vi "Simon_Mouse.vi"() -> ()   [LabVIEW 2019]
uses:
  <vilib>/numeric/Random Number (Range) U64.vi
  <vilib>/numeric/sub_Random U32.vi
  <vilib>/Utility/file.llb/Write Delimited Spreadsheet (I64).vi
panel:
  in  "读档":bool
  in  "存档":bool
  in  "亮灯次数":i32=1
  out "难度：分数":string
  out "倒计时":i32(slide) scale=-1.0..3635.0
  in  "是否开始计时？":bool
  out "分数":i32
  out "难度":string="困难"
  out "闪烁间隔":i32=727
  out "超时时间":i32=500
  out "User name out":string
  in  "User name in":string
  in  "结束":bool
  out "时间到":bool
  out "上":bool
  out "左":bool
  out "右":bool
  out "下":bool
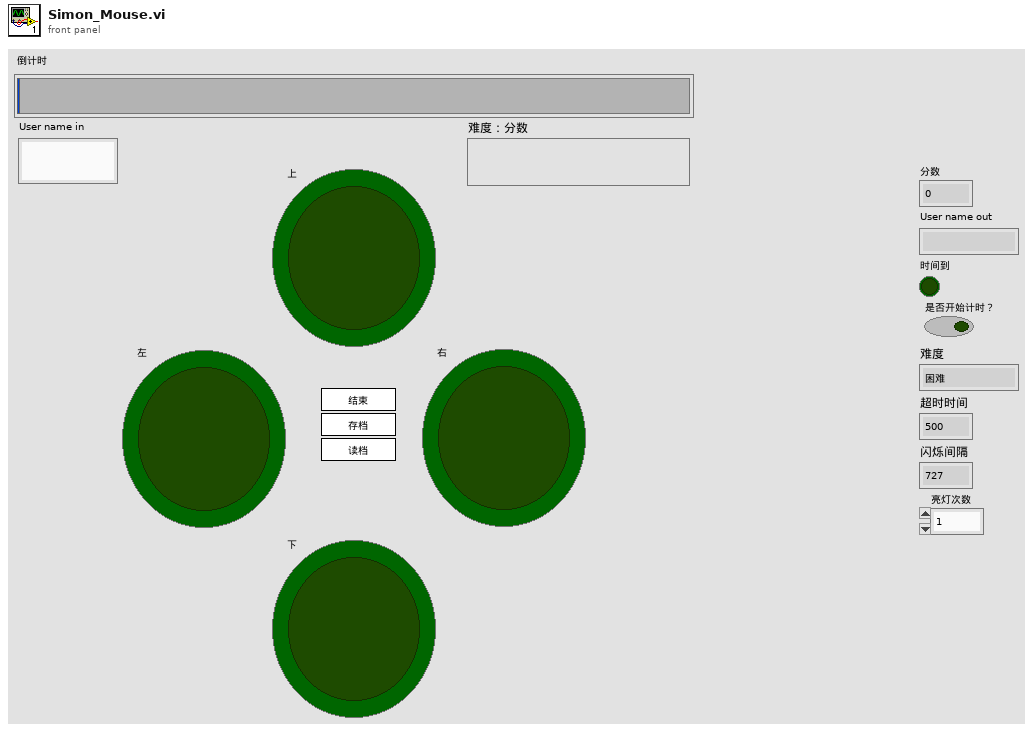
[diagram p1: front panel]
types:
  T1 = enum32{"Invalid", "Standard", "Closed", "Hidden", "Minimized", "Maximized"}
  T2 = enum32{"invalid app kind", "Development System", "Run Time System", "Student Edition", "Embedded LabVIEW", "Evaluation", "Custom"}
  T3 = typedef "按键枚举.ctl" = enum16{"读档", "存档", "按错", "退出", "黄", "红", "蓝", "绿"}
  T4 = cluster{"Core":cluster{"Current VI Reference":refnum<vi>, "Close Panel on Exit?":bool, "难度_保存":string, "亮灯次数_保存":i32, "超时时间_保存":i32, "闪烁间隔_保存":i32, "积分_保存":i32}}
  T5 = cluster{"Current VI Reference":refnum<vi>, "Close Panel on Exit?":bool, "难度_保存":string, "亮灯次数_保存":i32, "超时时间_保存":i32, "闪烁间隔_保存":i32, "积分_保存":i32}
  T6 = enum16{"Left Button", "Center Button", "Right Button", "Window Close"}
  T7 = typedef "eventvkey.ctl" = enum16{"ASCII", "Enter", "Return", "Shift", "Ctrl", "Alt", "Cmd", "Opt", "Caps", "NumLock", "Clear", "Break", "Up", "Down", "Left", "Right", "Insert", "Delete", "Home", "End", "PageUp", "PageDown", "Escape", "Help", "Pause", "ScrollLock", "F1", "F2", "F3", "F4", "F5", "F6", "F7", "F8", "F9", "F10", "F11", "F12", "F13", "F14", "F15", "F16", "F17", "F18", "F19", "F20", "F21", "F22", "F23", "F24", "Play", "VolumeUp", "VolumeDown", "Mute", "Two Byte Char"}
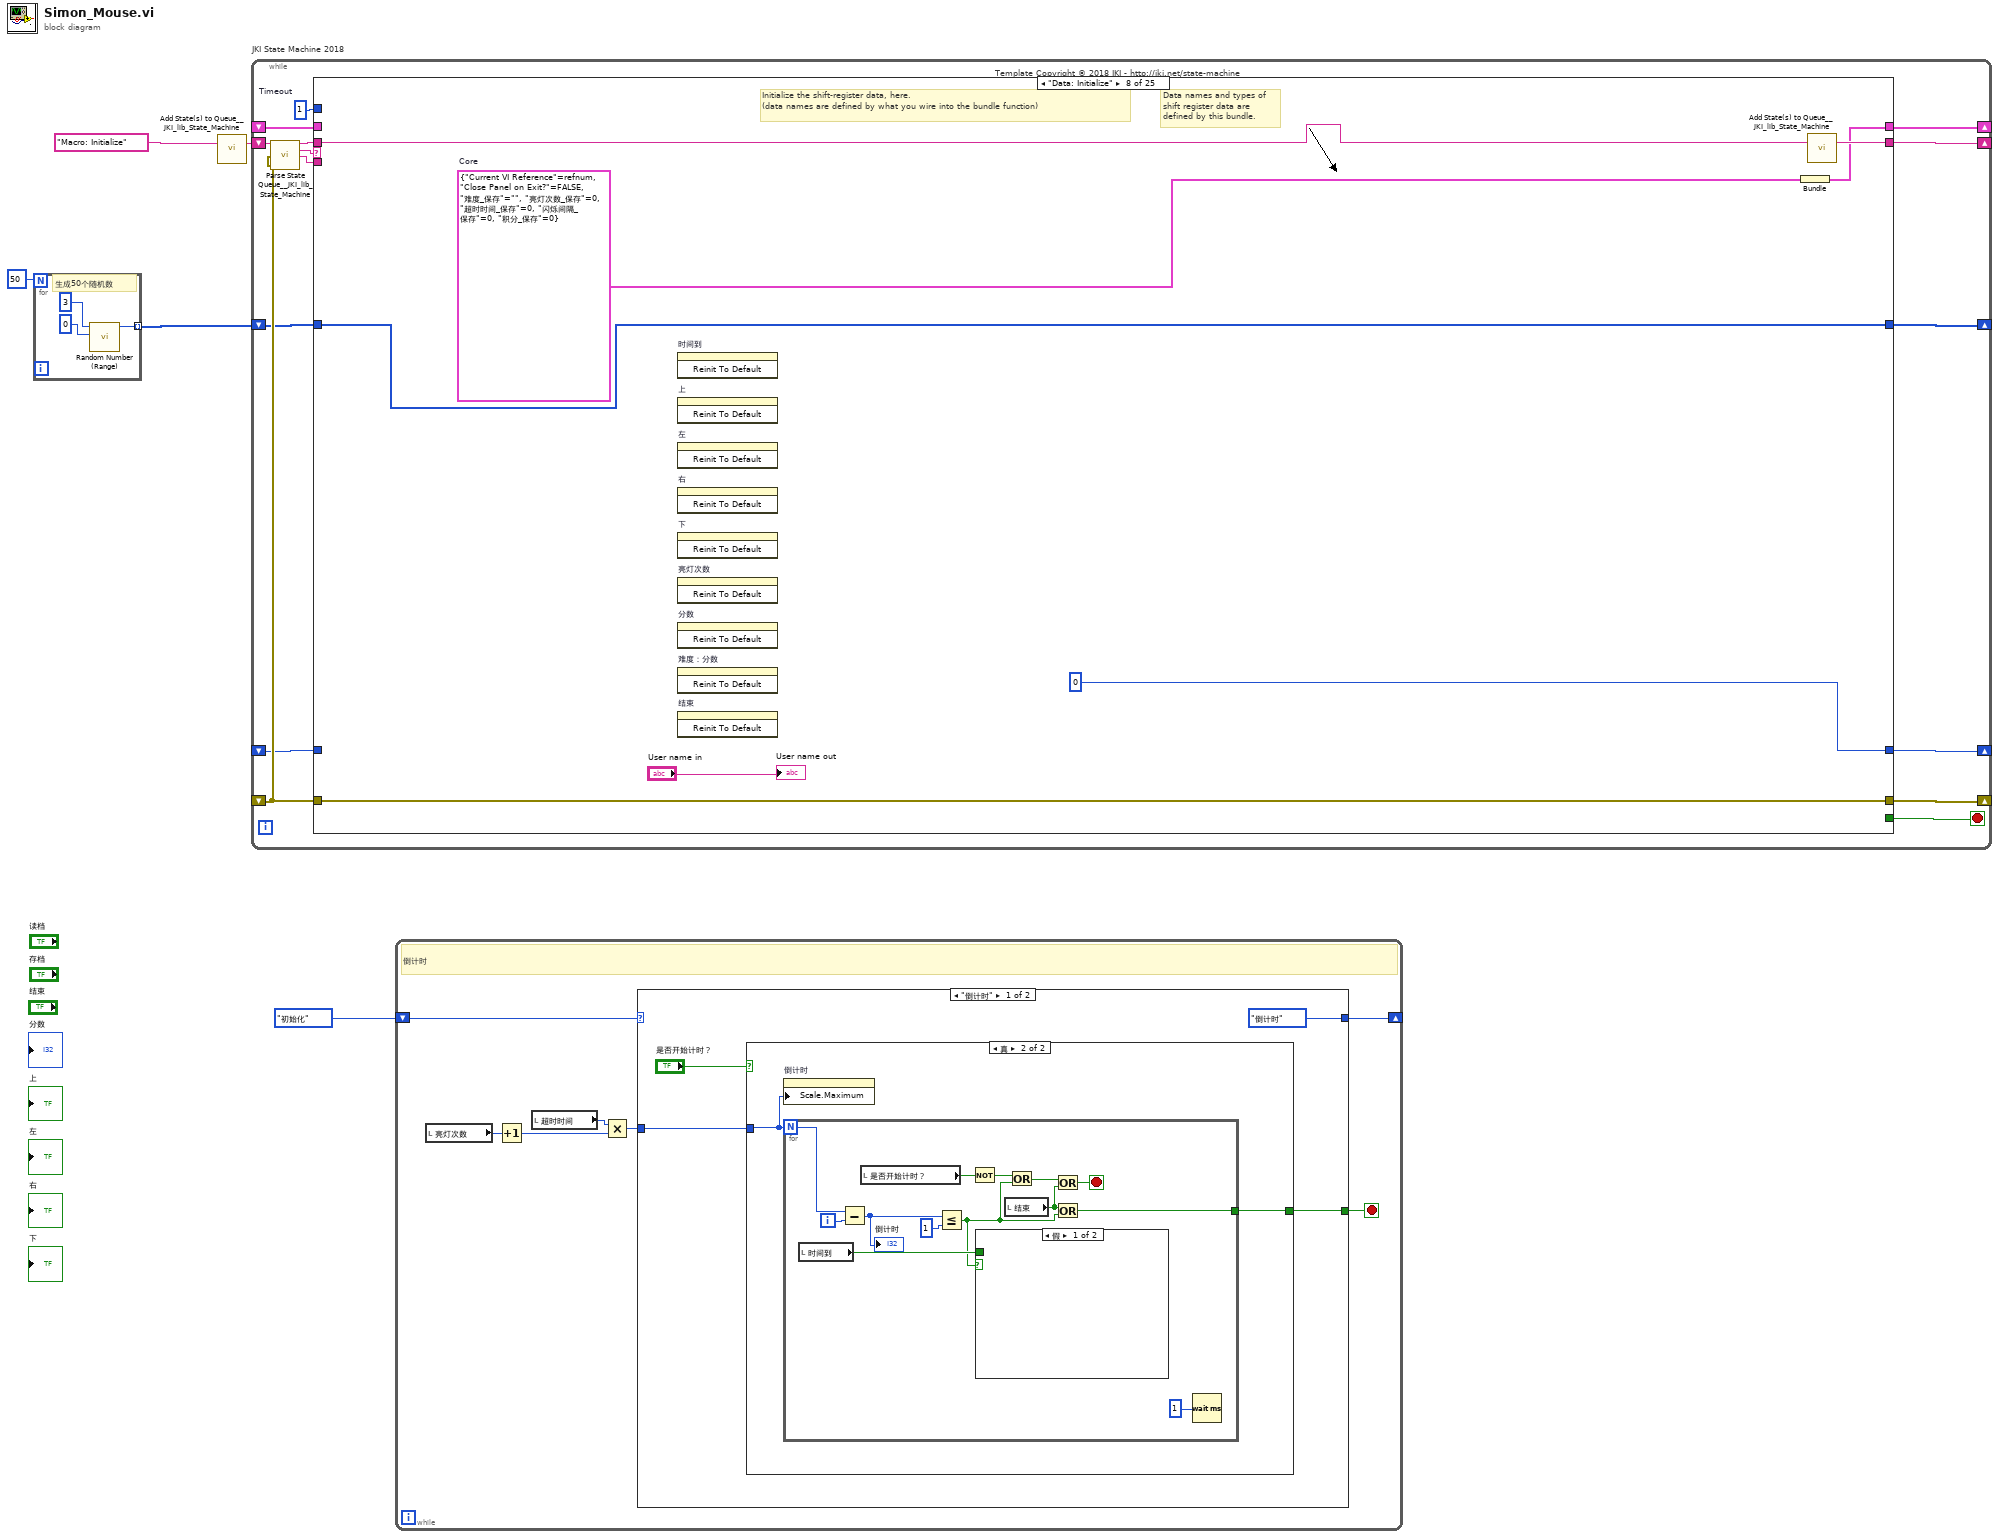
[diagram p0: block diagram]
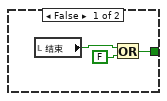
[diagram p2: hidden frame]
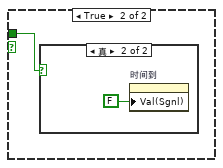
[diagram p3: hidden frame]
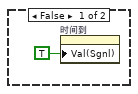
[diagram p4: hidden frame]
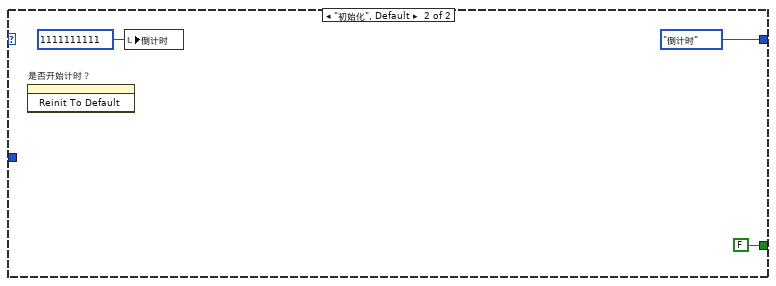
[diagram p5: hidden frame]
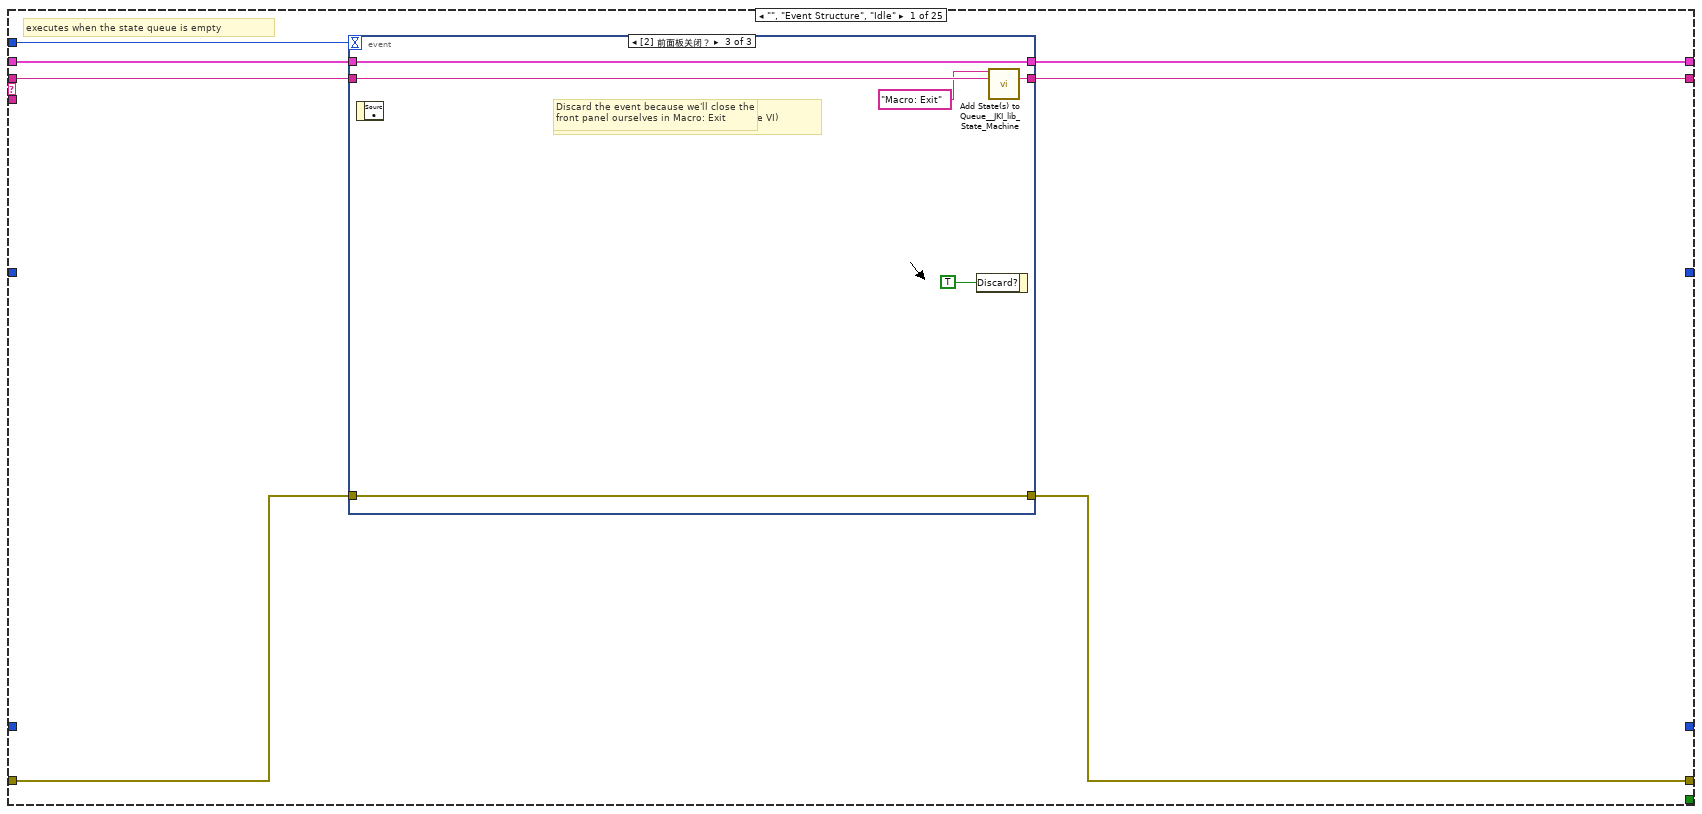
[diagram p6: hidden frame]
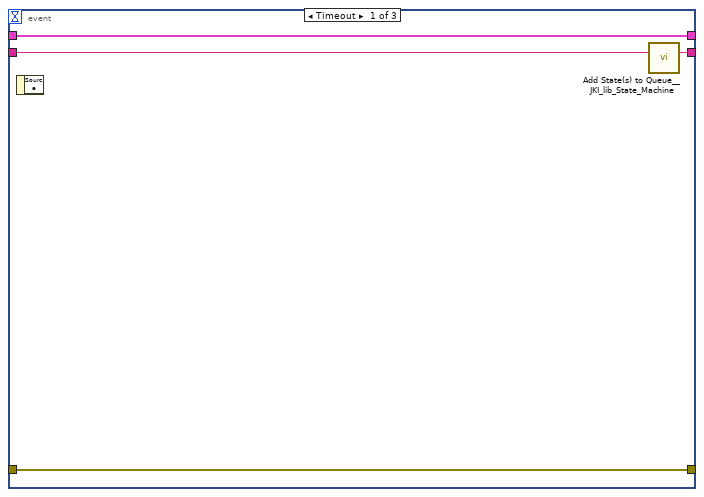
[diagram p7: hidden frame]
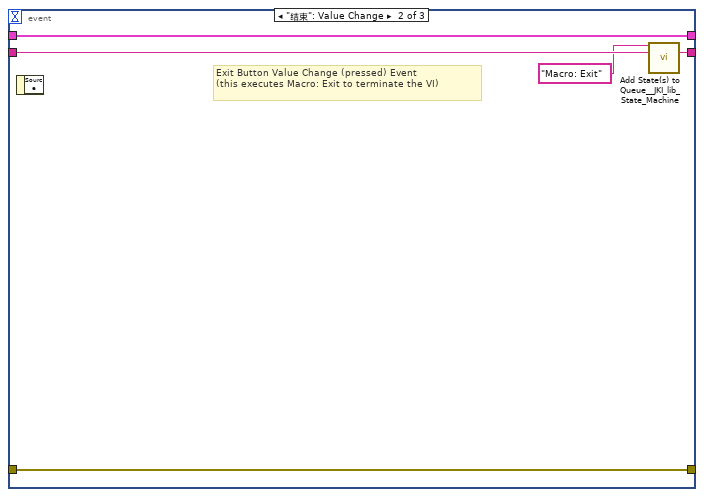
[diagram p8: hidden frame]
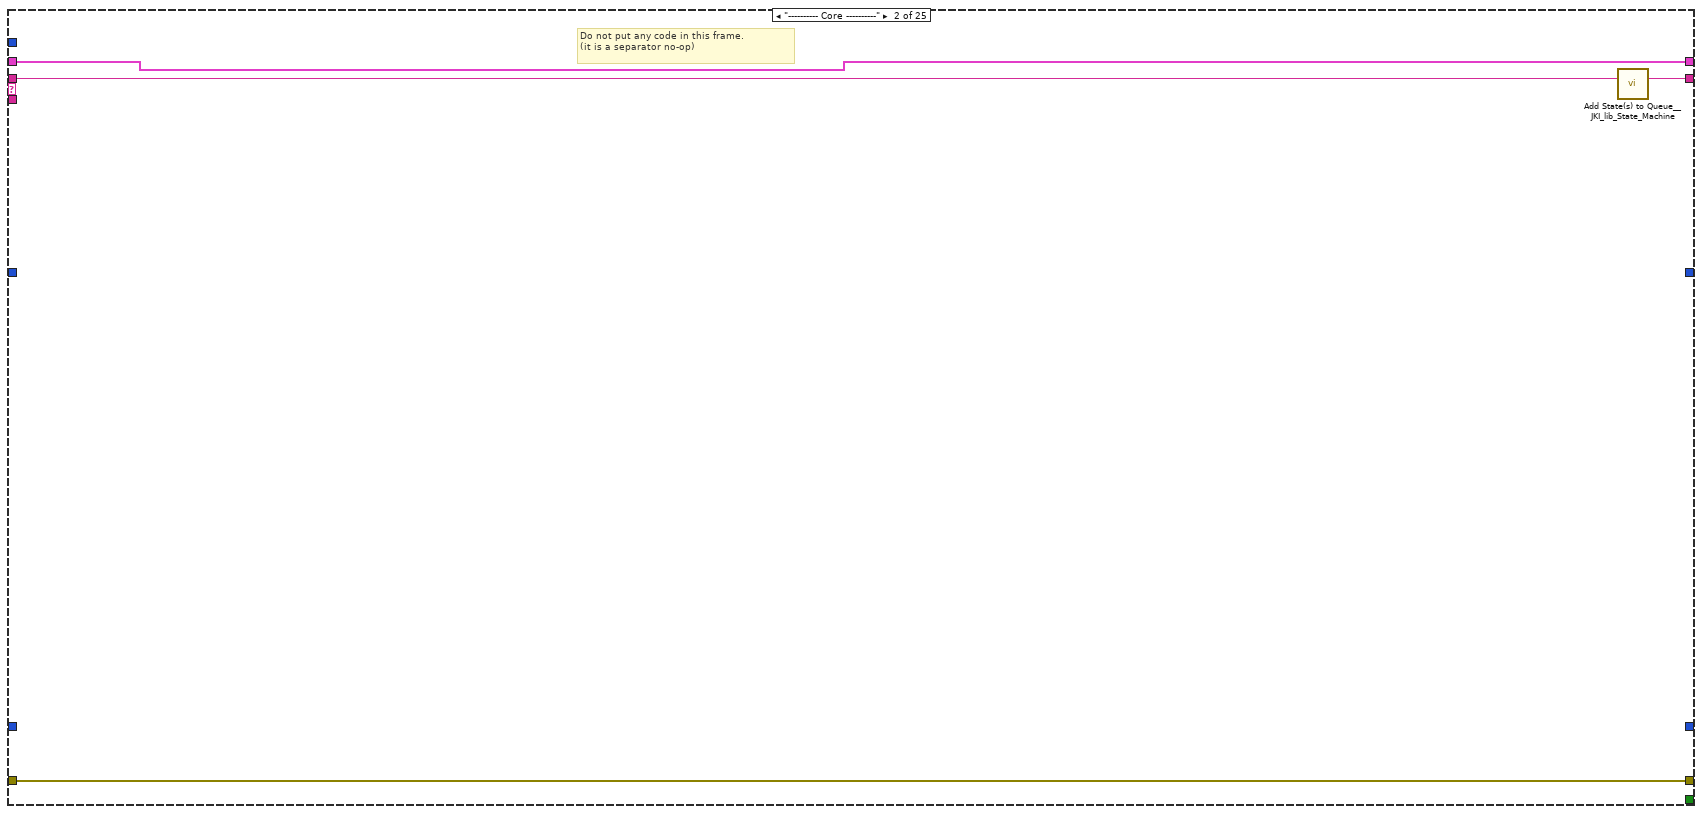
[diagram p9: hidden frame]
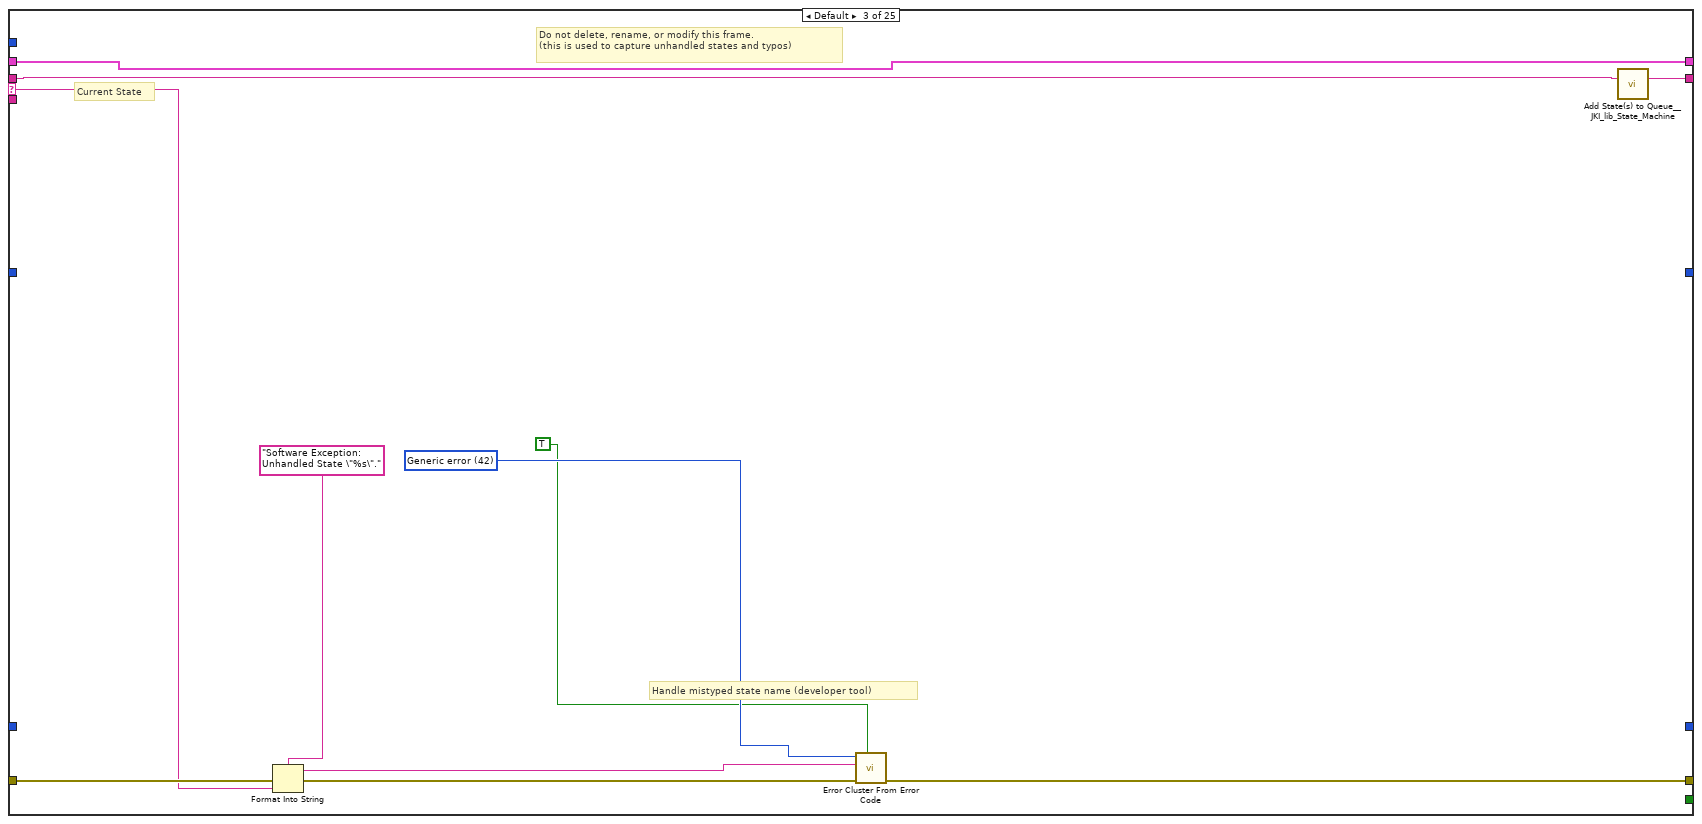
[diagram p10: hidden frame]
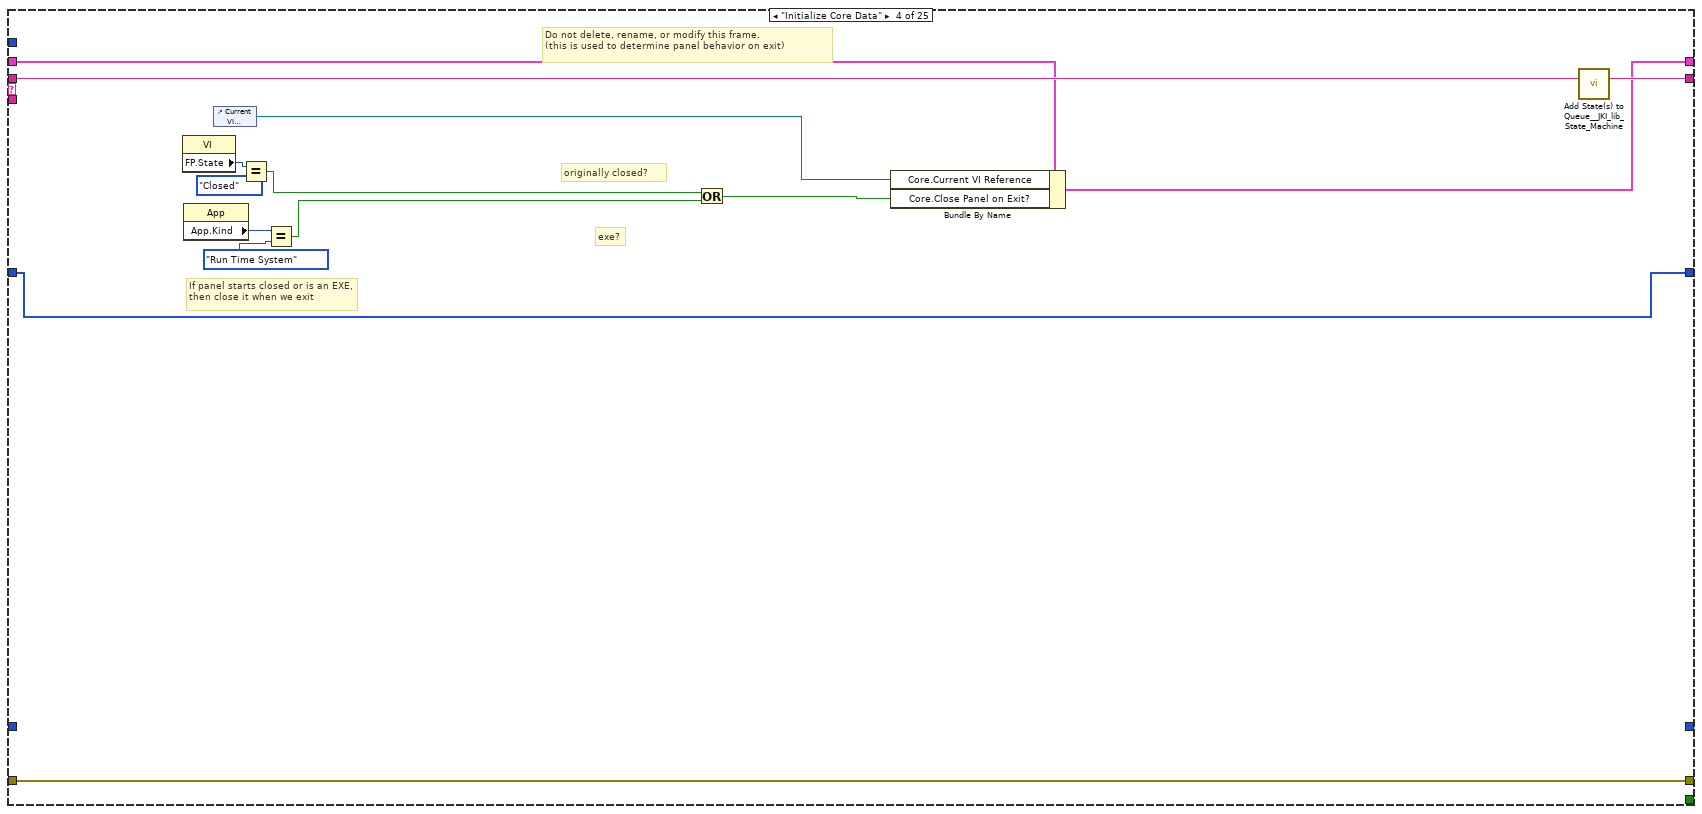
[diagram p11: hidden frame]
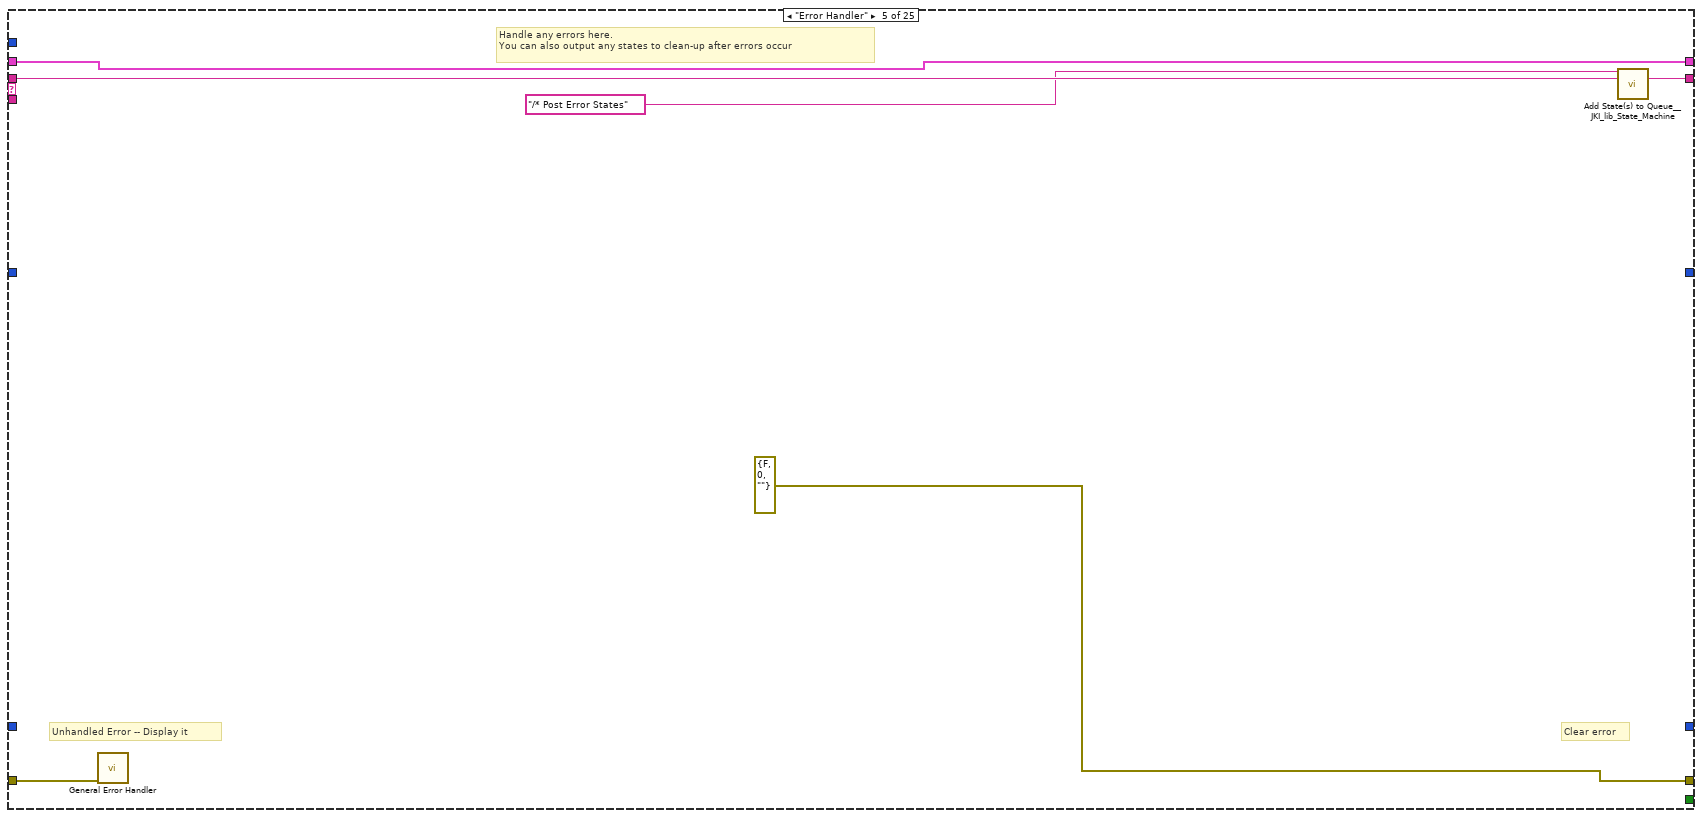
[diagram p12: hidden frame]
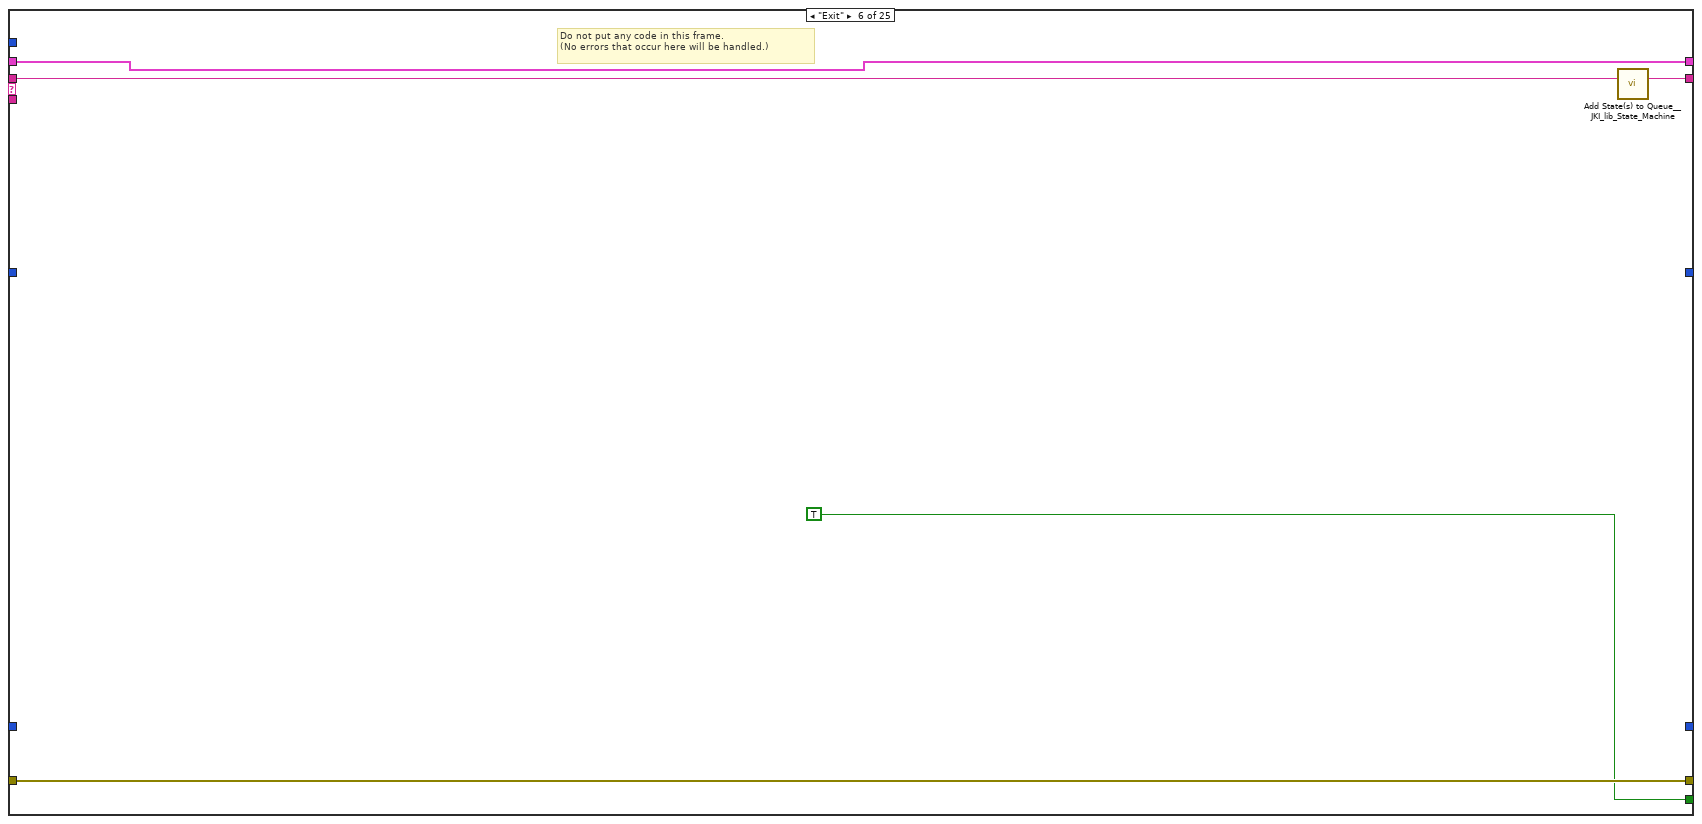
[diagram p13: hidden frame]
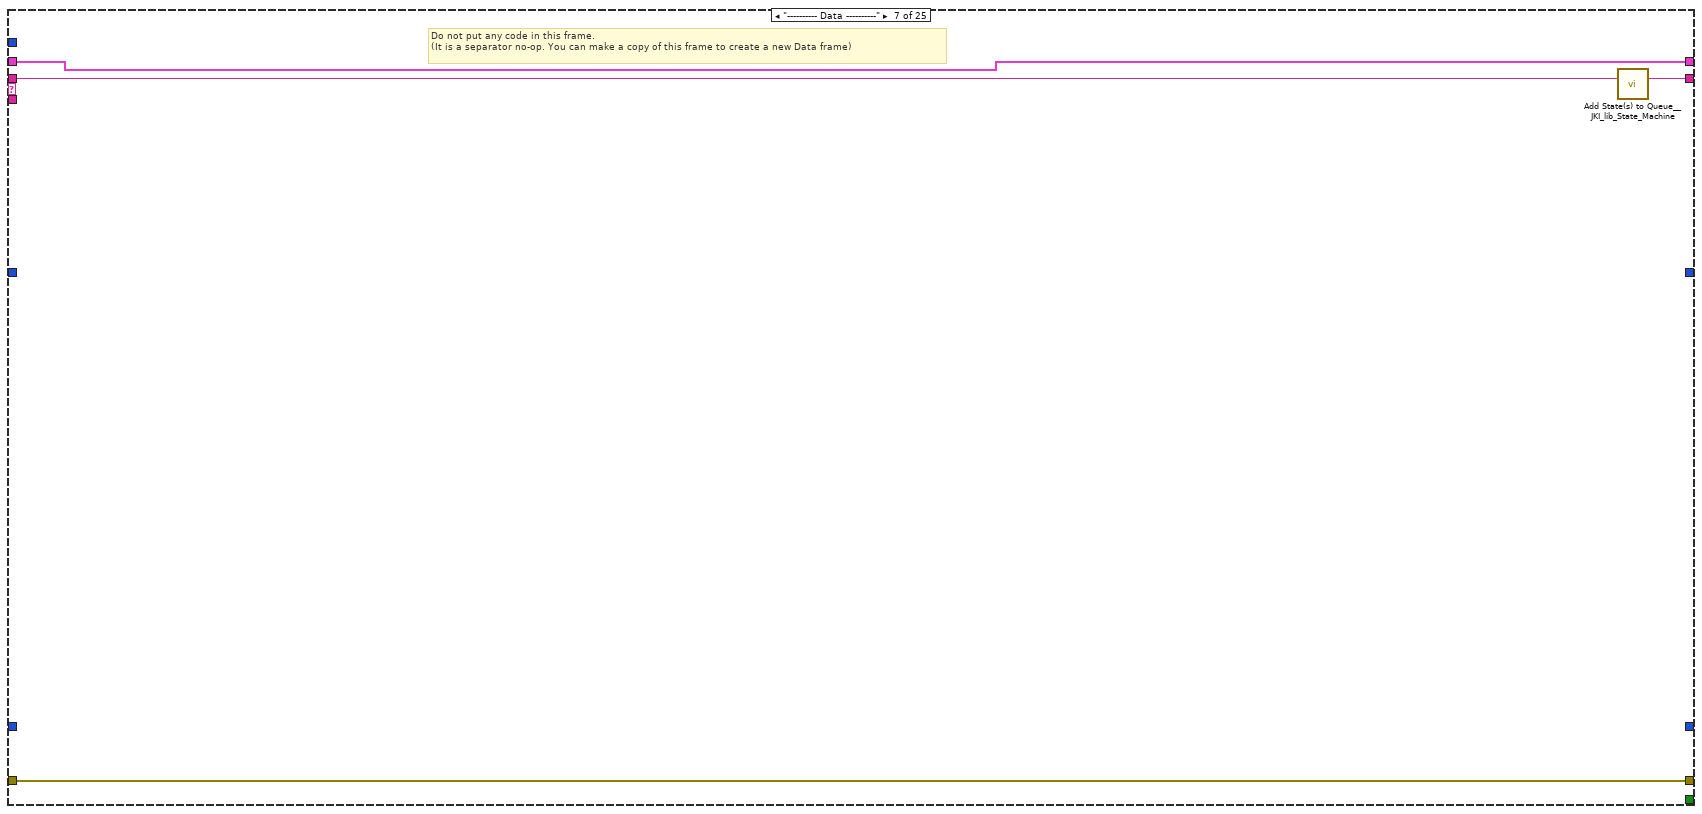
[diagram p14: hidden frame]
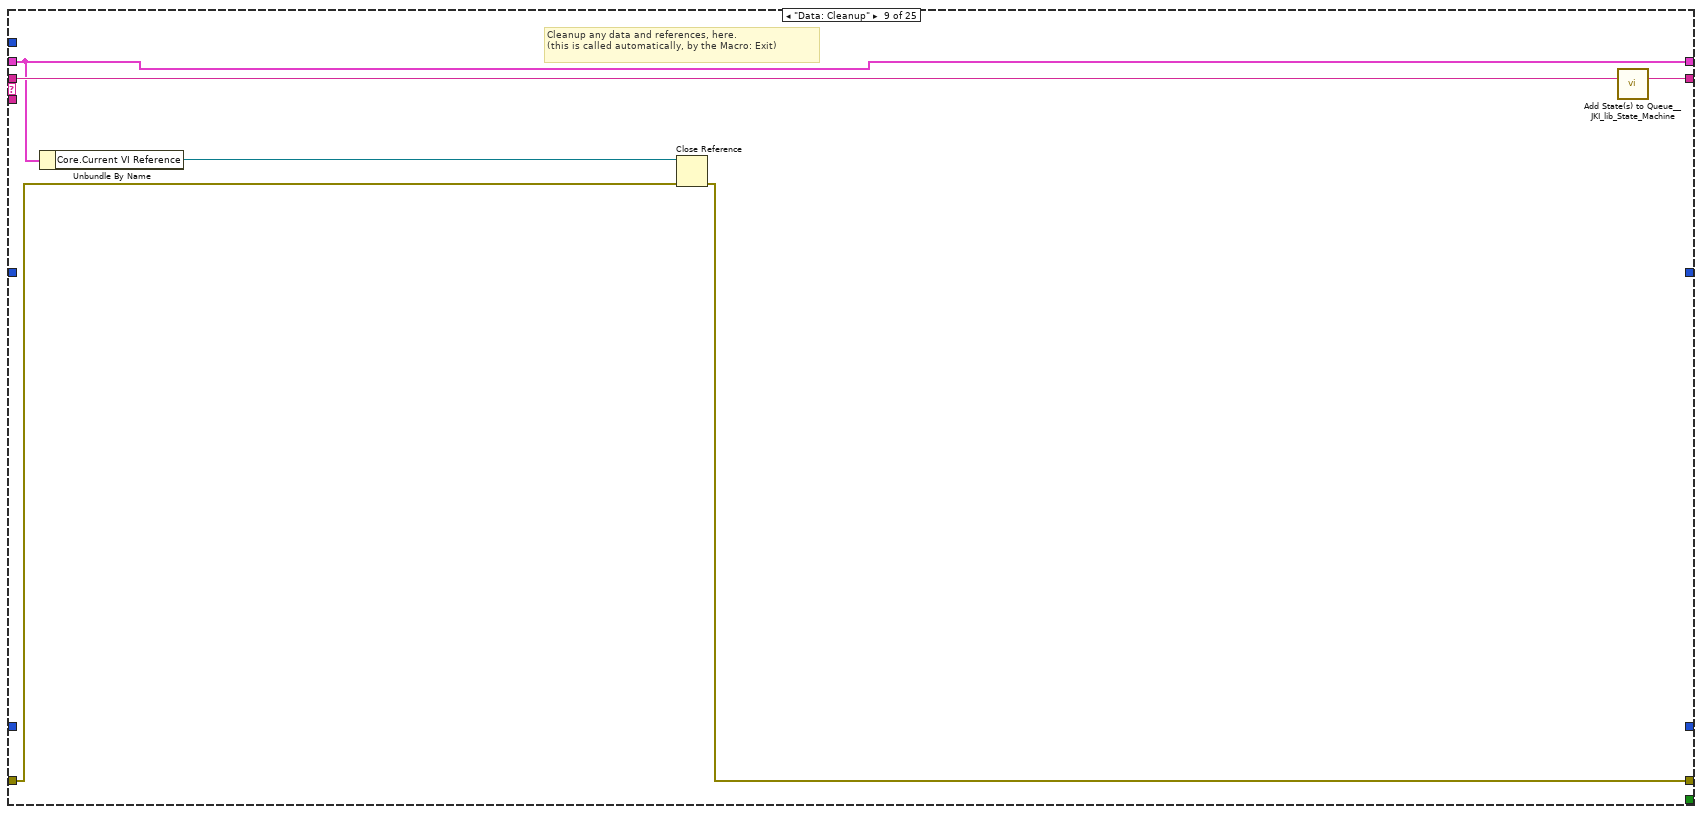
[diagram p15: hidden frame]
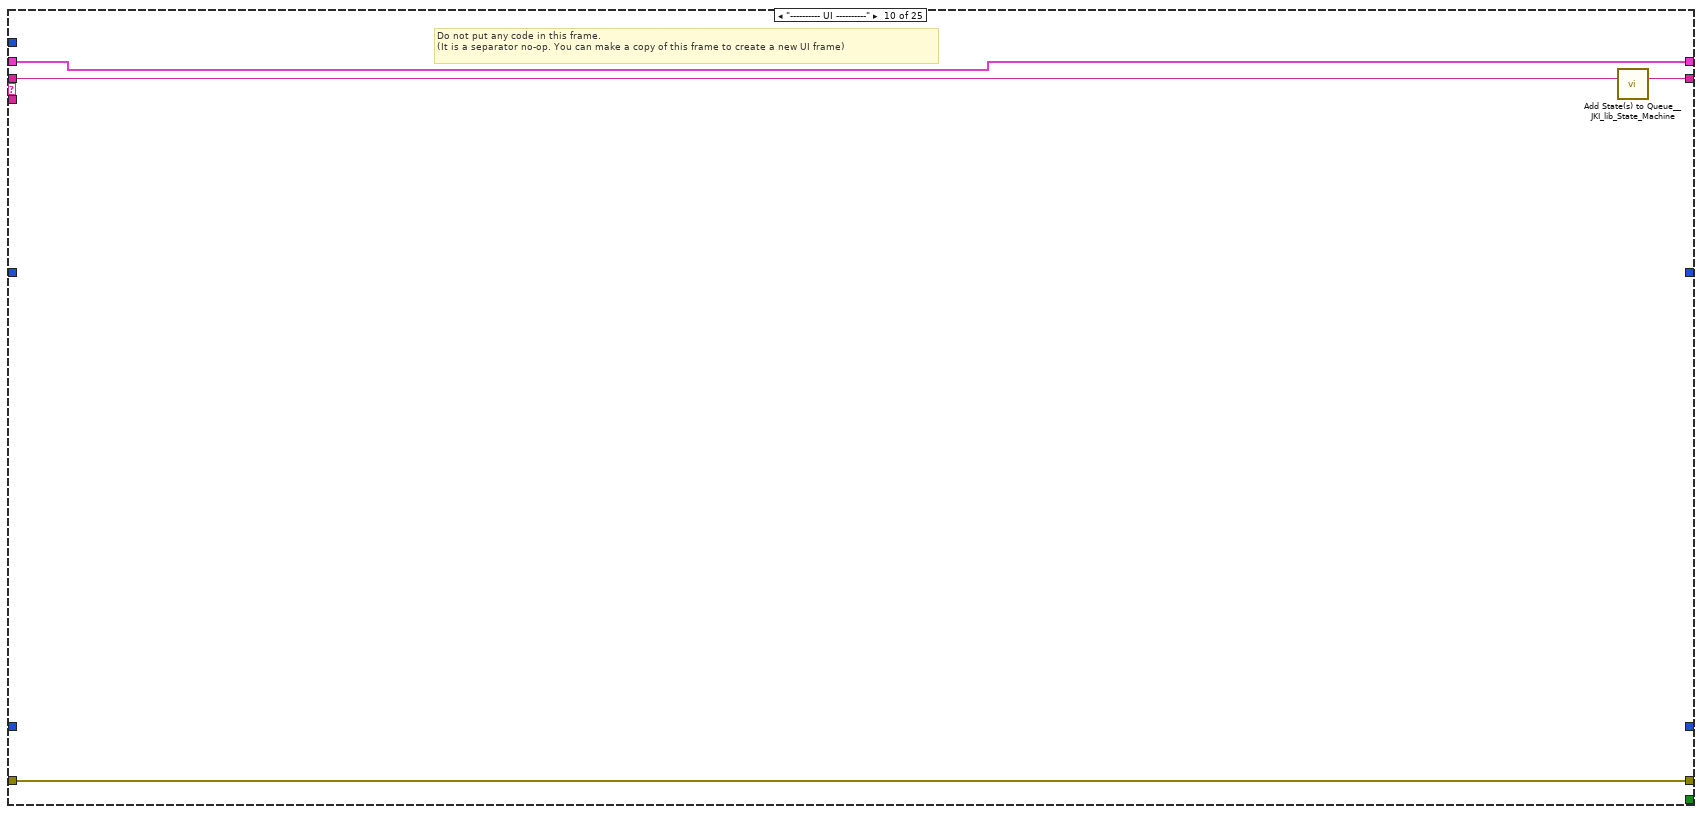
[diagram p16: hidden frame]
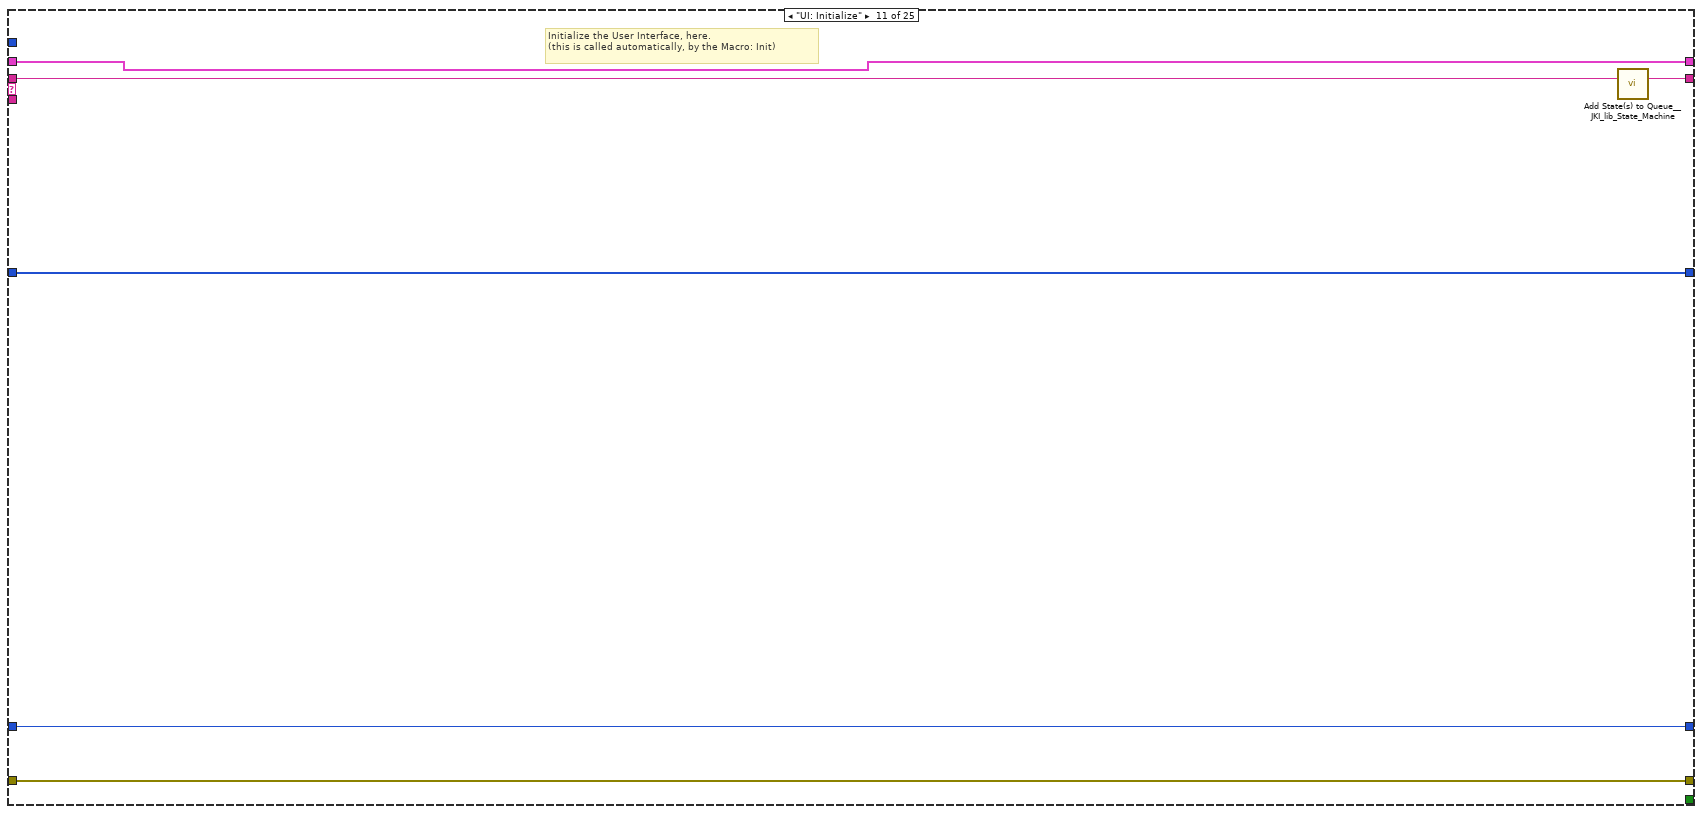
[diagram p17: hidden frame]
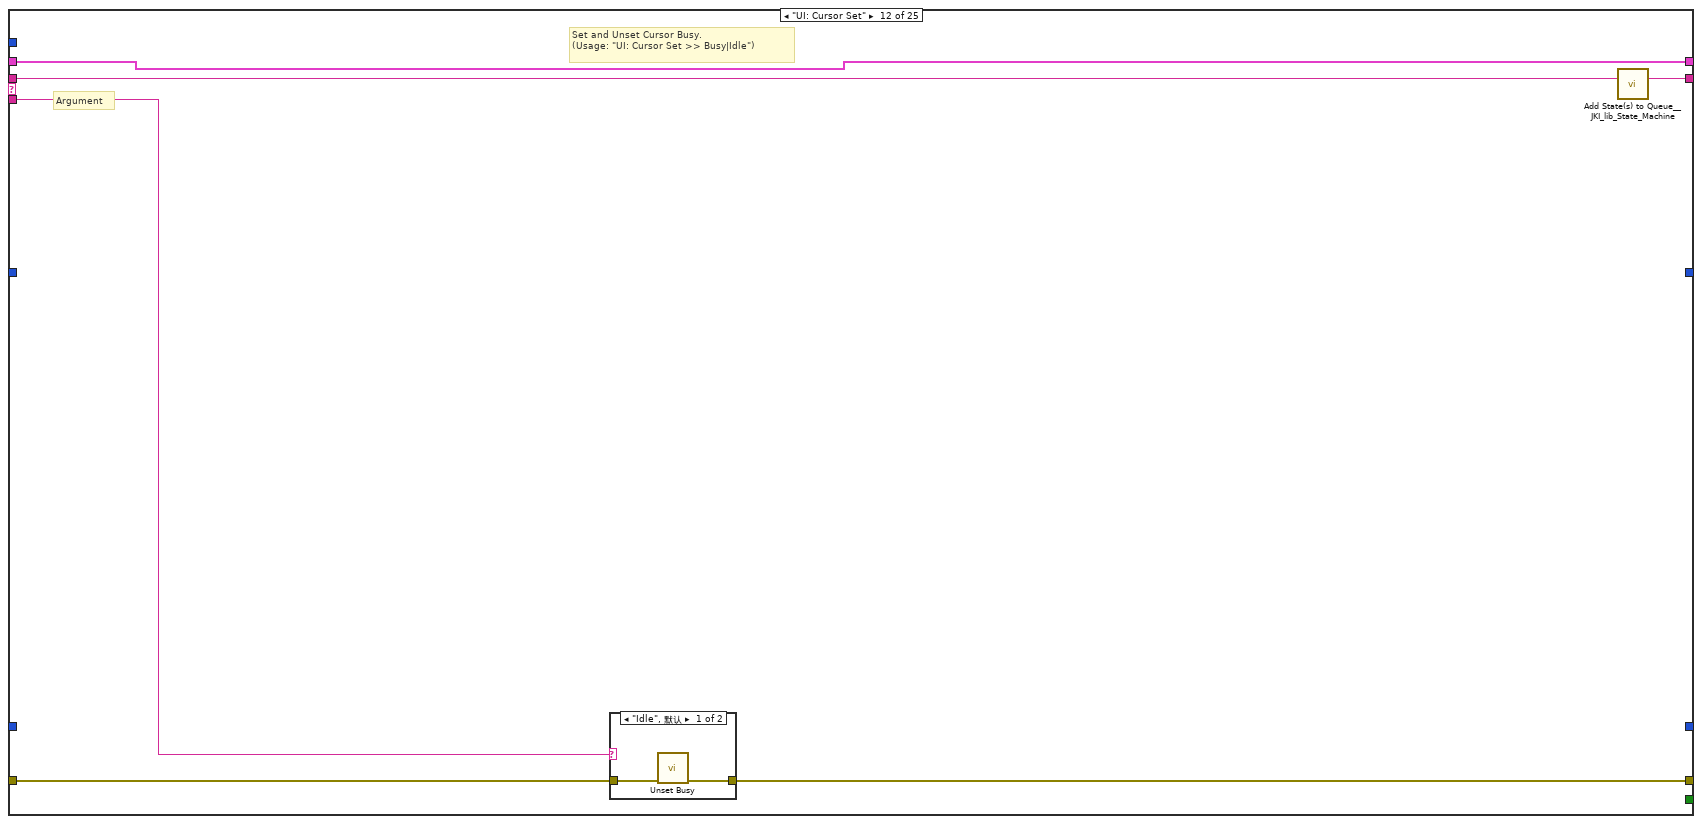
[diagram p18: hidden frame]
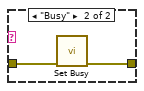
[diagram p19: hidden frame]
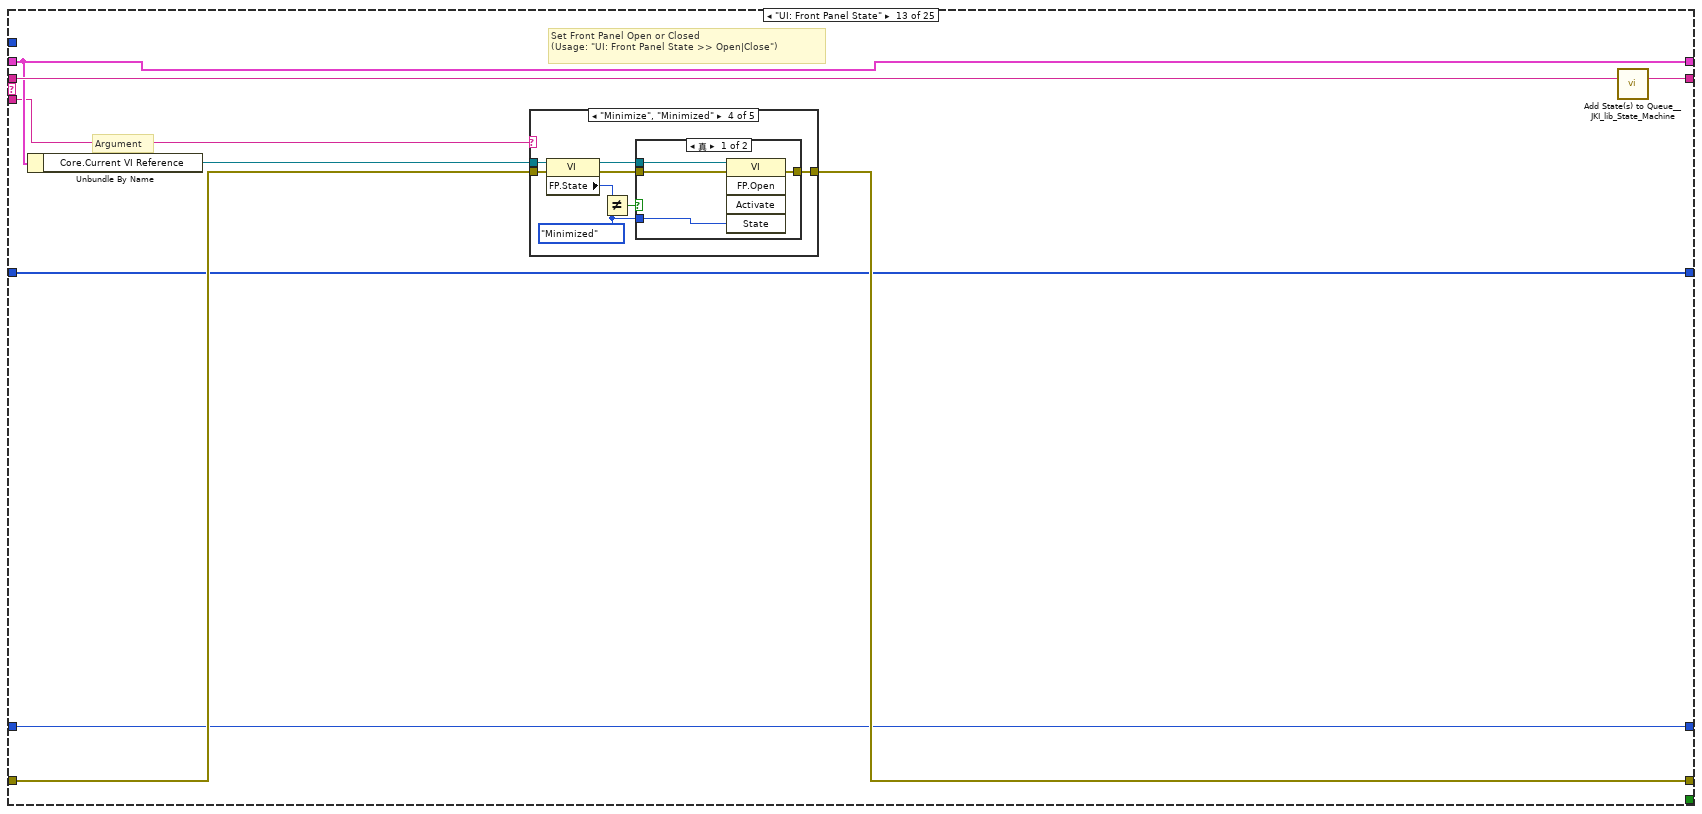
[diagram p20: hidden frame]
diagram:
  n1 = for {
    N: 50 -> [_]
    tunnel: [w6] -> w2 mode=indexing
    # "生成50个随机数"
    n2 = call-poly <vilib>:"Random Number (Range).vi"("lower bound (0)"=u64 0, "upper bound (100)"=u64 3) -> ("number"=w6:u64)  [unwired: 9 in]
  }
  n3 = call <vilib>:"Add State(s) to Queue__JKI_lib_State_Machine.vi"("State(s) in (\"\")"="Macro: Initialize") -> ("States Out"=w5:string)  [unwired: 14 in]
  n4 = while "JKI State Machine 2018" {
    shift-right: [w16] -> _
    shift-left: _ -> [w15]
    shift-right: [w19] -> _
    shift-left: _ -> [w13]
    shift-right: [w18] -> _
    shift-left: w5 -> [w20]
    shift-right: [w12] -> _
    shift-left: w2 -> [w11]
    shift-right: [w9] -> _
    shift-left: _ -> [w10]
    stop <- w17 stop-if-true
    w14 = 1  # Timeout
    # "Template Copyright © 2018 JKI - http://jki.net/state-machine"
    n5 = call <vilib>:"Parse State Queue__JKI_lib_State_Machine.vi"("State Queue"=w20, "Error In (no error)"=w13) -> ("Remaining States"=w22:string, "Current State"=w23:string, "Arguments"=w21:string)  [unwired: 11 in]
    n6 = case shown="\"Data: Initialize\"" w23 {
      selector: w23 -> [_ _ w50 _ _ _ _ _ _ _ _ _ _ _ _ _ _ _ _ _ _ _ _ _ _]
      tunnel: w22 -> [w30 w49 w54 w74 w80 w85 w89 w97 w103 w107 w113 w119 w132 w201 w208 w218 w222 w226 w244 w267 w286 w312 w330 w460 w481]
      tunnel: w21 -> [_ _ _ _ _ _ _ _ _ _ _ w114 w126 _ _ _ _ _ _ _ _ _ _ _ _]
      tunnel: w15 -> [w28 w46 w52 w67 w77 w83 w86 _ w98 w104 w108 w117 w128 w198 w205 w215 w219 w223 w241 w252 w277 w309 w327 w457 w468]
      tunnel: [w27 w47 w56 w71 errorcluster {"status"=FALSE, "code"=0, "source"=""} ("error out") w82 w87 w94 w99 w105 w111 w115 w129 w199 w206 w216 w220 w224 w242 w265 w284 w310 w328 w458 w479] -> w19
      tunnel: w13 -> [w26 w47 w55 w71 w76 w82 w87 w94 w100 w105 w111 w116 w130 w199 w206 w216 w220 w224 w242 w265 w284 w310 w328 w458 w479]
      tunnel: [w29 w48 w53 w73 w79 w84 w88 w96 w102 w106 w112 w118 w131 w200 w207 w217 w221 w225 w243 w266 w285 w311 w329 w459 w480] -> w18
      tunnel: [_ _ _ _ _ TRUE _ _ _ _ _ _ _ _ _ _ _ _ _ _ _ _ _ TRUE _] -> w17
      tunnel: [w25 w46 w52 w72 w77 w83 w86 w95 w98 w104 w108 w117 w128 w198 w205 w215 w219 w223 w241 w251 w277 w309 w327 w457 w467] -> w16
      tunnel: w14 -> [w24 _ _ _ _ _ _ _ _ _ _ _ _ _ _ _ _ _ _ _ _ _ _ _ _]
      tunnel: [_ _ _ w61 _ _ _ w92 _ _ w110 _ w125 _ w203 _ _ _ w236 w255 w283 w308 w315 w456 w478] -> w12
      tunnel: w11 -> [_ _ _ w61 _ _ _ w92 _ _ w110 _ w125 _ w203 _ _ _ w236 w255 w283 w308 w315 w456 w478]
      tunnel: [_ _ _ _ _ _ _ 0 _ _ w109 _ w124 _ w202 _ _ _ w227 w254 w279 1 w322 w453 w469] -> w9
      tunnel: w10 -> [_ _ _ _ _ _ _ _ _ _ w109 _ w124 _ w202 _ _ _ w227 w254 w279 _ w314 w453 w469]
      frame "", "Event Structure", "Idle" {
        # "executes when the state queue is empty"
        n7 = event shown="[2] 前面板关闭？" {
          selector: _ -> [_ _ _]
          dyn-events: _ -> [_ _ _]
          timeout: w24 -> [_ _ _]
          tunnel: w30 -> [w34 w39 w45]
          tunnel: [w33 w38 w44] -> w29
          tunnel: w28 -> [w31 w36 w42]
          tunnel: [w32 w37 w43] -> w27
          tunnel: w26 -> [w32 w37 w43]
          tunnel: [w31 w36 w42] -> w25
          event Timeout {
            n8 = event-data() -> ()  [unwired: 1 in, 1 out]
            n9 = call <vilib>:"Add State(s) to Queue__JKI_lib_State_Machine.vi"("State(s) in (\"\")"=w34) -> ("States Out"=w33:string)  [unwired: 14 in]
          }
          event "结束": Value Change {
            # "Exit Button Value Change (pressed) Event\n(this executes Macro: Exit to terminate the VI)"
            n10 = event-data() -> ()  [unwired: 1 in, 1 out]
            n11 = call <vilib>:"Add State(s) to Queue__JKI_lib_State_Machine.vi"("State(s) in Front (\"\")"="Macro: Exit", "State(s) in (\"\")"=w39) -> ("States Out"=w38:string)  [unwired: 13 in]
          }
          event Panel Close? {
            # "Discard the event because we'll close the front panel ourselves in Macro: Exit"
            # "Close Panel button (pressed) Event\n(this executes Macro: Exit to terminate the VI)"
            n12 = event-data() -> ()  [unwired: 1 in, 1 out]
            n13 = event-data("Discard?"=TRUE) -> ()  [unwired: 1 in, 1 out]
            n14 = call <vilib>:"Add State(s) to Queue__JKI_lib_State_Machine.vi"("State(s) in Front (\"\")"="Macro: Exit", "State(s) in (\"\")"=w45) -> ("States Out"=w44:string)  [unwired: 13 in]
          }
        }
      }
      frame "---------- Core ----------" {
        # "Do not put any code in this frame.\n(it is a separator no-op)"
        n15 = call <vilib>:"Add State(s) to Queue__JKI_lib_State_Machine.vi"("State(s) in (\"\")"=w49) -> ("States Out"=w48:string)  [unwired: 14 in]
      }
      frame Default {
        w59 = 42 items=["No error", "Argument error", "Memory is full", "Out of zone", "End of file", "File already open", "Generic file I/O error", "File not found", "File permission error", "Disk is full", "Duplicate path", "Too many files open", "System feature not enabled", "Resource file not found", "Cannot add resource", "Resource not found", "Image not found", "Image memory error", "Pen does not exist", "Config type invalid", "Config token not found", "Config parse error", "Config memory error", "Bad external code format", "Bad external code offset", "External code not present", "Null window", "Destroy window error", "Null menu", "Print aborted", "Bad print record", "Print driver error", "Windows error during printing", "Memory error during printing", "Print dialog error", "Generic print error", "Invalid device refnum", "Device not found", "Device parameter error", "Device unit error", "Cannot open device", "Device call aborted", "Generic error", "Cancelled by user", "Object ID too low", "Object ID too high", "Object not in heap", "Unknown heap", "Unknown object (invalid DefProc)", "Unknown object (DefProc not in table)", "Message out of range", "Invalid (null) method", "Unknown message", "Manager call not supported", "Bad address", "Network operation in progress", "Network operation timed out", "Connection is busy", "Network attribute not supported", "Network error", "Address in use", "System out of memory", "Connection aborted", "Connection refused", "Not connected", "Already connected", "Connection closed", "Initialization error (interapplication manager)", "Bad occurrence", "Wait on unbound occurrence handler", "Occurrence queue overflow", "Datalog type conflict", "Unused", "Unrecognized type (interapplication manager)", "Memory corrupt", "Failed to make temporary DLL", "Old CIN version", "Drag socket not found", "Failed to load drop-object", "Failed to register OLE object", "Failed to release OLE object", "Format specifier type mismatch", "Unknown format specifier", "Too few format specifiers", "Too many format specifiers", "Scan failed", "Newer CIN version", "Error converting to variant", "Runtime menu error", "Password tampered", "Variant attribute not found", "Incompatible variant data type", "Event data is not available", "Event Store is not present", "Occurrence is not found", "Event Queue is not created", "Event info is not available", "Refnum passed is NULL", "Error retrieving Class GUID", "Error retrieving CoClass GUID", "Error retrieving TypeLib GUID.", "Bad built application magic bytes.", "Specific driver is different from the specific driver associated with the Logical Name.", "There is no session opened to the class driver.", "Max Error", "MAX - Error with config objects", "MAX - Error loading configuration", "MAX - Group not supported"]
        # "Current State"
        # "Do not delete, rename, or modify this frame.\n(this is used to capture unhandled states and typos)"
        # "Handle mistyped state name (developer tool)"
        n16 = Format Into String(format string="Software Exception: Unhandled State \"%s\"." ("message"), error in=w55, w50) -> (resulting string=w58:string, error out=w57:errorcluster)  [unwired: 1 in]
        n17 = call <vilib>:"Error Cluster From Error Code.vi"("show call chain? (False)"=TRUE, "error in (no error)"=w57, "error message (\"\")"=w58, "error code (0)"=w59) -> ("error out"=w56:errorcluster)  [unwired: 5 in]
        n18 = call <vilib>:"Add State(s) to Queue__JKI_lib_State_Machine.vi"("State(s) in (\"\")"=w54) -> ("States Out"=w53:string)  [unwired: 14 in]
      }
      frame "Initialize Core Data" {
        # "Do not delete, rename, or modify this frame.\n(this is used to determine panel behavior on exit)"
        # "originally closed?"
        # "exe?"
        # "If panel starts closed or is an EXE, then close it when we exit"
        n19 = property class="VI"() -> ("FP.State"=w64:T1)  [unwired: 2 in, 2 out]
        n20 = property class="App"() -> ("App.Kind"=w70:T2)  [unwired: 2 in, 2 out]
        n21 = control-ref of="Current VI Reference"() -> (w65:refnum<vi>)
        n22 = Equal?(x=w64, y=T1."Closed" ("Front Panel Window:State")) -> (x = y?=w62:bool)
        n23 = Equal?(x=w70, y=T2."Run Time System" ("Application:Kind")) -> (x = y?=w68:bool)
        n24 = Or(x=w62, y=w68) -> (x .or. y?=w66:bool)
        n25 = Bundle By Name(cluster=w67, "Core.Current VI Reference"=w65, "Core.Close Panel on Exit?"=w66) -> (w72:T4)
        n26 = call <vilib>:"Add State(s) to Queue__JKI_lib_State_Machine.vi"("State(s) in (\"\")"=w74) -> ("States Out"=w73:string)  [unwired: 14 in]
      }
      frame "Error Handler" {
        # "Unhandled Error -- Display it"
        # "Handle any errors here.\nYou can also output any states to clean-up after errors occur"
        # "Clear error"
        n27 = call <vilib>:"General Error Handler.vi"("error in (no error)"=w76) -> ()  [unwired: 10 in, 5 out]
        n28 = call <vilib>:"Add State(s) to Queue__JKI_lib_State_Machine.vi"("State(s) in Front (\"\")"="/* Post Error States", "State(s) in (\"\")"=w80) -> ("States Out"=w79:string)  [unwired: 13 in]
      }
      frame "Exit" {
        # "Do not put any code in this frame.\n(No errors that occur here will be handled.)"
        n29 = call <vilib>:"Add State(s) to Queue__JKI_lib_State_Machine.vi"("State(s) in (\"\")"=w85) -> ("States Out"=w84:string)  [unwired: 14 in]
      }
      frame "---------- Data ----------" {
        # "Do not put any code in this frame.\n(It is a separator no-op. You can make a copy of this frame to create a new Data frame)"
        n30 = call <vilib>:"Add State(s) to Queue__JKI_lib_State_Machine.vi"("State(s) in (\"\")"=w89) -> ("States Out"=w88:string)  [unwired: 14 in]
      }
      frame "Data: Initialize" {
        w90 = T5 {"Current VI Reference"=refnum, "Close Panel on Exit?"=FALSE, "难度_保存"="", "亮灯次数_保存"=0, "超时时间_保存"=0, "闪烁间隔_保存"=0, "积分_保存"=0}  # Core
        # "Data names and types of shift register data are defined by this bundle."
        # "Initialize the shift-register data, here.\n(data names are defined by what you wire into the bundle function)"
        n31 = invoke on="时间到" class="Bool (严格)" method="Reinit To Default"() -> ()  [unwired: 3 in, 3 out]
        n32 = invoke on="上" class="Bool (严格)" method="Reinit To Default"() -> ()  [unwired: 3 in, 3 out]
        n33 = invoke on="左" class="Bool (严格)" method="Reinit To Default"() -> ()  [unwired: 3 in, 3 out]
        n34 = invoke on="右" class="Bool (严格)" method="Reinit To Default"() -> ()  [unwired: 3 in, 3 out]
        n35 = invoke on="下" class="Bool (严格)" method="Reinit To Default"() -> ()  [unwired: 3 in, 3 out]
        n36 = invoke on="亮灯次数" class="DigNum (严格)" method="Reinit To Default"() -> ()  [unwired: 3 in, 3 out]
        n37 = invoke on="分数" class="DigNum (严格)" method="Reinit To Default"() -> ()  [unwired: 3 in, 3 out]
        n38 = invoke on="难度：分数" class="Str" method="Reinit To Default"() -> ()  [unwired: 3 in, 3 out]
        n39 = invoke on="结束" class="Bool (严格)" method="Reinit To Default"() -> ()  [unwired: 3 in, 3 out]
        n40 = Bundle("Core"=w90) -> (w95:T4)  [unwired: 1 in]
        n41 = call <vilib>:"Add State(s) to Queue__JKI_lib_State_Machine.vi"("State(s) in (\"\")"=w97) -> ("States Out"=w96:string)  [unwired: 14 in]
        "User name out" <- "User name in"
      }
      frame "Data: Cleanup" {
        # "Cleanup any data and references, here.\n(this is called automatically, by the Macro: Exit)"
        n42 = Unbundle By Name(w98) -> ("Core.Current VI Reference"=w101:refnum<vi>)
        n43 = Close Reference(reference=w101, error in (no error)=w100) -> (error out=w99:errorcluster)
        n44 = call <vilib>:"Add State(s) to Queue__JKI_lib_State_Machine.vi"("State(s) in (\"\")"=w103) -> ("States Out"=w102:string)  [unwired: 14 in]
      }
      frame "---------- UI ----------" {
        # "Do not put any code in this frame.\n(It is a separator no-op. You can make a copy of this frame to create a new UI frame)"
        n45 = call <vilib>:"Add State(s) to Queue__JKI_lib_State_Machine.vi"("State(s) in (\"\")"=w107) -> ("States Out"=w106:string)  [unwired: 14 in]
      }
      frame "UI: Initialize" {
        # "Initialize the User Interface, here.\n(this is called automatically, by the Macro: Init)"
        n46 = call <vilib>:"Add State(s) to Queue__JKI_lib_State_Machine.vi"("State(s) in (\"\")"=w113) -> ("States Out"=w112:string)  [unwired: 14 in]
      }
      frame "UI: Cursor Set" {
        # "Argument"
        # "Set and Unset Cursor Busy.\n(Usage: \"UI: Cursor Set >> Busy|Idle\")"
        n47 = case shown="\"Idle\", 默认" w114 {
          tunnel: w116 -> [w121 w123]
          tunnel: [w120 w122] -> w115
          frame "Idle", Default {
            n48 = call <vilib>:"Unset Busy.vi"("error in (no error)"=w121) -> ("error out"=w120:errorcluster)  [unwired: 10 in]
          }
          frame "Busy" {
            n49 = call <vilib>:"Set Busy.vi"("error in (no error)"=w123) -> ("error out"=w122:errorcluster)  [unwired: 9 in, 1 out]
          }
        }
        n50 = call <vilib>:"Add State(s) to Queue__JKI_lib_State_Machine.vi"("State(s) in (\"\")"=w119) -> ("States Out"=w118:string)  [unwired: 14 in]
      }
      frame "UI: Front Panel State" {
        # "Argument"
        # "Set Front Panel Open or Closed\n(Usage: \"UI: Front Panel State >> Open|Close\")"
        n51 = Unbundle By Name(w128) -> ("Core.Current VI Reference"=w127:refnum<vi>)
        n52 = case shown="\"Minimize\", \"Minimized\"" w126 {
          tunnel: w130 -> [w138 w153 w164 w177 w190]
          tunnel: [w140 w154 w166 w179 w192] -> w129
          tunnel: w127 -> [w139 w151 w165 w178 w191]
          frame "Open", "Standard", Default {
            w133 = T1."Standard" ("State")
            n53 = property class="VI"(reference=w139, error in=w138) -> (reference out=w136:refnum<vi>, error out=w137:errorcluster, "FP.State"=w135:T1)
            n54 = Not Equal?(x=w135, y=w133) -> (x != y?=w134:bool)
            n55 = case shown="假" w134 {
              tunnel: [w144 w146] -> w140
              tunnel: w137 -> [w143 w146]
              tunnel: w136 -> [w142 _]
              tunnel: w133 -> [w141 _]
              frame True {
                n56 = invoke class="VI" method="FP.Open"(reference=w142, error in=w143, "Activate"=TRUE, "State"=w141) -> (error out=w144:errorcluster)  [unwired: 1 in, 4 out]
              }
              frame False {
              }
            }
          }
          frame "Close", "Closed" {
            n57 = property class="VI"(reference=w151, error in=w153) -> (reference out=w150:refnum<vi>, error out=w152:errorcluster, "FP.State"=w148:T1)
            n58 = Not Equal?(x=w148, y=T1."Closed" ("Front Panel Window:State")) -> (x != y?=w147:bool)
            n59 = case shown="真" w147 {
              tunnel: [w155 w158] -> w154
              tunnel: w152 -> [w155 w157]
              tunnel: w150 -> [_ w156]
              frame False {
              }
              frame True {
                n60 = invoke class="VI" method="FP.Close"(reference=w156, error in=w157) -> (error out=w158:errorcluster)  [unwired: 1 in, 2 out]
              }
            }
          }
          frame "Hidden", "Hide" {
            w159 = T1."Hidden" ("State")
            n61 = property class="VI"(reference=w165, error in=w164) -> (reference out=w162:refnum<vi>, error out=w163:errorcluster, "FP.State"=w161:T1)
            n62 = Not Equal?(x=w161, y=w159) -> (x != y?=w160:bool)
            n63 = case shown="真" w160 {
              tunnel: [w170 w171] -> w166
              tunnel: w163 -> [w169 w171]
              tunnel: w162 -> [w168 _]
              tunnel: w159 -> [w167 _]
              frame True {
                n64 = invoke class="VI" method="FP.Open"(reference=w168, error in=w169, "State"=w167) -> (error out=w170:errorcluster)  [unwired: 2 in, 4 out]
              }
              frame False {
              }
            }
          }
          frame "Minimize", "Minimized" {
            w172 = T1."Minimized" ("State")
            n65 = property class="VI"(reference=w178, error in=w177) -> (reference out=w175:refnum<vi>, error out=w176:errorcluster, "FP.State"=w174:T1)
            n66 = Not Equal?(x=w174, y=w172) -> (x != y?=w173:bool)
            n67 = case shown="真" w173 {
              tunnel: [w183 w184] -> w179
              tunnel: w176 -> [w182 w184]
              tunnel: w175 -> [w181 _]
              tunnel: w172 -> [w180 _]
              frame True {
                n68 = invoke class="VI" method="FP.Open"(reference=w181, error in=w182, "State"=w180) -> (error out=w183:errorcluster)  [unwired: 2 in, 4 out]
              }
              frame False {
              }
            }
          }
          frame "Maximize", "Maximized" {
            w185 = T1."Maximized" ("State")
            n69 = property class="VI"(reference=w191, error in=w190) -> (reference out=w188:refnum<vi>, error out=w189:errorcluster, "FP.State"=w187:T1)
            n70 = Not Equal?(x=w187, y=w185) -> (x != y?=w186:bool)
            n71 = case shown="真" w186 {
              tunnel: [w196 w197] -> w192
              tunnel: w189 -> [w195 w197]
              tunnel: w188 -> [w194 _]
              tunnel: w185 -> [w193 _]
              frame True {
                n72 = invoke class="VI" method="FP.Open"(reference=w194, error in=w195, "State"=w193) -> (error out=w196:errorcluster)  [unwired: 2 in, 4 out]
              }
              frame False {
              }
            }
          }
        }
        n73 = call <vilib>:"Add State(s) to Queue__JKI_lib_State_Machine.vi"("State(s) in (\"\")"=w132) -> ("States Out"=w131:string)  [unwired: 14 in]
      }
      frame "---------- Macro ----------" {
        # "Do not put any code in this frame.\n(It is a separator no-op. You can make a copy of this frame to create a new Macro frame)"
        n74 = call <vilib>:"Add State(s) to Queue__JKI_lib_State_Machine.vi"("State(s) in (\"\")"=w201) -> ("States Out"=w200:string)  [unwired: 14 in]
      }
      frame "Macro: Initialize" {
        w204 = "Data: Initialize\nInitialize Core Data\nUI: Initialize\nUI: Front Panel State >> Open\nGame: Select difficulty"  # Data: Initialize Initialize Core Data UI: Initialize UI: Front Panel State >> Open Game: Select difficulty
        # "Initialization Macro\n(This is called once, when the VI starts)"
        n75 = call <vilib>:"Add State(s) to Queue__JKI_lib_State_Machine.vi"("State(s) in Front (\"\")"=w204, "State(s) in (\"\")"=w208) -> ("States Out"=w207:string)  [unwired: 13 in]
      }
      frame "Macro: Exit" {
        # "Exit Macro\n(This is called once, when the VI exits)"
        n76 = Unbundle By Name(w215) -> ("Core.Close Panel on Exit?"=w214:bool)
        n77 = Select(t="UI: Front Panel State >> Close", s=w214, f="") -> (s? t:f=w211:string)
        n78 = call <vilib>:"Add State(s) to Queue__JKI_lib_State_Machine.vi"("State(s) in (\"\")"=w211, "State(s) at Back (\"\")"="Data: Cleanup\nExit") -> ("States Out"=w209:string)  [unwired: 13 in]
        n79 = call <vilib>:"Add State(s) to Queue__JKI_lib_State_Machine.vi"("State(s) in Front (\"\")"=w209, "State(s) in (\"\")"=w218) -> ("States Out"=w217:string)  [unwired: 13 in]
      }
      frame "---------- Game ----------" {
        # "Template Separator\n(You can make a copy of, or modify, this frame)"
        n80 = call <vilib>:"Add State(s) to Queue__JKI_lib_State_Machine.vi"("State(s) in (\"\")"=w222) -> ("States Out"=w221:string)  [unwired: 14 in]
      }
      frame "Game: Read" {
        # "Template Separator\n(You can make a copy of, or modify, this frame)"
        n81 = call <vilib>:"Add State(s) to Queue__JKI_lib_State_Machine.vi"("State(s) in (\"\")"=w226) -> ("States Out"=w225:string)  [unwired: 14 in]
      }
      frame "Game: Save" {
        # "Template Separator\n(You can make a copy of, or modify, this frame)"
        n82 = Unbundle By Name(w241) -> ("Core.难度_保存"=w234:string, "Core.亮灯次数_保存"=w239:i32, "Core.超时时间_保存"=w238:i32, "Core.闪烁间隔_保存"=w237:i32, "Core.积分_保存"=w233:i32)
        n83 = case shown="\"困难\", 默认" w234 {
          tunnel: [2 0 1] -> w240
          frame "困难", Default {
          }
          frame "简单" {
          }
          frame "中等" {
          }
        }
        n84 = local write "是否开始计时？"(FALSE ("是否开始计时？")) -> ()
        n85 = Build Array(w240, w239, w238, w237, w233) -> (w235:i32[])
        n86 = Build Array(w236, w235) -> (w231:u64[][])
        n87 = call "文件对话框"("default name"="请选择表格") -> ("selected path"=w230:path)  [unwired: 11 in, 3 out]
        n88 = call-poly <vilib>:"Write Delimited Spreadsheet.vi"("file path (dialog if empty)"=w230, "2D data"=w231) -> ()  [unwired: 12 in, 2 out]
        n89 = call <vilib>:"Add State(s) to Queue__JKI_lib_State_Machine.vi"("State(s) in (\"\")"=w244, "State(s) at Back (\"\")"="Game: Option" ("State(s) at Back (\"\")")) -> ("States Out"=w243:string)  [unwired: 13 in]
      }
      frame "Game: Select difficulty" {
        # "Your code here.\n(You can make a copy of, or modify, this frame)"
        n90 = Concatenate Strings("欢迎" ("message"), "选择难度" ("string"), "\r") -> (w258:string)
        n91 = call <vilib>:"Three Button Dialog.vi"("Allow user to close window? (TRUE)"=FALSE, "Right Button Text (\"Cancel\")"="困难" ("Right Button Text (\"Cancel\")"), "Center Button Text (\"No\")"="中等" ("Center Button Text (\"No\")"), "Left Button Text (\"Yes\")"="简单" ("Left Button Text (\"Yes\")"), "message"=w258) -> ("Which Button?"=w256:T6)  [unwired: 6 in]
        n92 = case shown="\"Right Button\"" w256 {
          tunnel: [727 484 303] -> w248
          tunnel: [750 550 350] -> w249
          tunnel: ["简单" "中等" "困难"] -> w250
          frame "Left Button", Default {
          }
          frame "Center Button" {
          }
          frame "Right Button" {
          }
        }
        "超时时间" <- w248
        "闪烁间隔" <- w249
        "难度" <- w250
        n93 = Bundle By Name(cluster=w252, "Core.难度_保存"=w250, "Core.闪烁间隔_保存"=w249, "Core.超时时间_保存"=w248) -> (w251:T4)
        n94 = call <vilib>:"Add State(s) to Queue__JKI_lib_State_Machine.vi"("State(s) in (\"\")"=w267, "State(s) at Back (\"\")"="Game: Twinkle" ("State(s) at Back (\"\")")) -> ("States Out"=w266:string)  [unwired: 13 in]
      }
      frame "Game: Twinkle" {
        # "根据回合选择亮灯顺序"
        # "Your code here.\n(You can make a copy of, or modify, this frame)"
        n95 = Array Subset(array=w283, index=0 ("索引"), length="亮灯次数") -> (w281:u64[])
        n96 = for {
          tunnel: w281 -> [w287] mode=indexing
          stop <- w288 stop-if-true
          n97 = case shown="3" w287 {
            frame 0, Default {
              n98 = stacked-sequence {
                frame #0 {
                  n99 = local write "上"(TRUE) -> ()
                }
                frame #1 {
                  n100 = local read "闪烁间隔"() -> (w290:i32)
                  n101 = Wait (ms)(milliseconds to wait=w290) -> ()  [unwired: 1 out]
                }
                frame #2 {
                  n102 = local write "上"(FALSE) -> ()
                }
                frame #3 {
                  n103 = Wait (ms)(milliseconds to wait=u32 250 ("等待时间（毫秒）")) -> ()  [unwired: 1 out]
                }
              }
            }
            frame 1 {
              n104 = stacked-sequence {
                frame #0 {
                  n105 = local write "右"(TRUE) -> ()
                }
                frame #1 {
                  n106 = local read "闪烁间隔"() -> (w294:i32)
                  n107 = Wait (ms)(milliseconds to wait=w294) -> ()  [unwired: 1 out]
                }
                frame #2 {
                  n108 = local write "右"(FALSE) -> ()
                }
                frame #3 {
                  n109 = Wait (ms)(milliseconds to wait=u32 250 ("等待时间（毫秒）")) -> ()  [unwired: 1 out]
                }
              }
            }
            frame 2 {
              n110 = stacked-sequence {
                frame #0 {
                  n111 = local write "下"(TRUE) -> ()
                }
                frame #1 {
                  n112 = local read "闪烁间隔"() -> (w298:i32)
                  n113 = Wait (ms)(milliseconds to wait=w298) -> ()  [unwired: 1 out]
                }
                frame #2 {
                  n114 = local write "下"(FALSE) -> ()
                }
                frame #3 {
                  n115 = Wait (ms)(milliseconds to wait=u32 250 ("等待时间（毫秒）")) -> ()  [unwired: 1 out]
                }
              }
            }
            frame 3 {
              n116 = stacked-sequence {
                frame #0 {
                  n117 = local write "左"(TRUE) -> ()
                }
                frame #1 {
                  n118 = local read "闪烁间隔"() -> (w302:i32)
                  n119 = Wait (ms)(milliseconds to wait=w302) -> ()  [unwired: 1 out]
                }
                frame #2 {
                  n120 = local write "左"(FALSE) -> ()
                }
                frame #3 {
                  n121 = Wait (ms)(milliseconds to wait=u32 250 ("等待时间（毫秒）")) -> ()  [unwired: 1 out]
                }
              }
            }
          }
          n122 = local read "结束"() -> (w288:bool)
        }
        n123 = call <vilib>:"Add State(s) to Queue__JKI_lib_State_Machine.vi"("State(s) in (\"\")"=w286, "State(s) at Back (\"\")"="Game: start counting" ("State(s) at Back (\"\")")) -> ("States Out"=w285:string)  [unwired: 13 in]
      }
      frame "Game: start counting" {
        # "Template Separator\n(You can make a copy of, or modify, this frame)"
        n124 = local write "是否开始计时？"(TRUE ("是否开始计时？")) -> ()
        n125 = call <vilib>:"Add State(s) to Queue__JKI_lib_State_Machine.vi"("State(s) in (\"\")"=w312, "State(s) at Back (\"\")"="Game: Option" ("State(s) at Back (\"\")")) -> ("States Out"=w311:string)  [unwired: 13 in]
      }
      frame "Game: Option" {
        # "判断是否按完"
        # "判断是否超时"
        # "判断点亮的灯是否正确\n+1使判断的索引每循环一次向后移一位"
        # "鼠标点击与按键响应"
        # "提取要判断的灯号"
        # "Template Separator\n(You can make a copy of, or modify, this frame)"
        n126 = Decrement(x=w314) -> (x-1=w324:i32)
        n127 = Index Array(array=w315, index=w324) -> (element=w325:u64)
        n128 = event shown="[4] \"存档\": 鼠标按下" {
          selector: _ -> [_ _ _ _ _ _ _ _ _ _]
          dyn-events: _ -> [_ _ _ _ _ _ _ _ _ _]
          timeout: 10000 -> [_ _ _ _ _ _ _ _ _ _]
          tunnel: [按键枚举."绿" 按键枚举."退出" w394 按键枚举."红" 按键枚举."存档" 按键枚举."读档" 按键枚举."蓝" 按键枚举."黄" 按键枚举."按错" 按键枚举."退出"] -> w326
          tunnel: w314 -> [w386 w392 w393 w418 w424 w426 w428 w434 w440 w443]
          tunnel: [w386 w392 w393 w418 w424 w426 w428 w434 w440 w443] -> w323
          event "上": Mouse Down {
            n129 = event-data() -> ()  [unwired: 1 in, 8 out]
            n130 = stacked-sequence {
              frame #0 {
                n131 = local write "上"(TRUE ("上")) -> ()
              }
              frame #1 {
                n132 = Wait (ms)(milliseconds to wait=u32 60 ("等待时间（毫秒）")) -> ()  [unwired: 1 out]
              }
              frame #2 {
                n133 = local write "上"(FALSE ("上")) -> ()
              }
              frame #3 {
                n134 = Wait (ms)(milliseconds to wait=u32 60 ("等待时间（毫秒）")) -> ()  [unwired: 1 out]
              }
            }
          }
          event "结束": Value Change {
            n135 = event-data() -> ()  [unwired: 1 in, 6 out]
          }
          event Key Down {
            n136 = event-data() -> ("VKey"=w395:T7)  [unwired: 1 in, 7 out]
            n137 = case shown="\"ASCII\", 默认" w395 {
              tunnel: [按键枚举."按错" 按键枚举."绿" 按键枚举."蓝" 按键枚举."红" 按键枚举."黄"] -> w394
              frame "ASCII", Default {
              }
              frame "Up" {
                n138 = stacked-sequence {
                  frame #0 {
                    n139 = local write "上"(TRUE ("上")) -> ()
                  }
                  frame #1 {
                    n140 = Wait (ms)(milliseconds to wait=u32 60 ("等待时间（毫秒）")) -> ()  [unwired: 1 out]
                  }
                  frame #2 {
                    n141 = local write "上"(FALSE ("上")) -> ()
                  }
                  frame #3 {
                    n142 = Wait (ms)(milliseconds to wait=u32 60 ("等待时间（毫秒）")) -> ()  [unwired: 1 out]
                  }
                }
              }
              frame "Right" {
                n143 = stacked-sequence {
                  frame #0 {
                    n144 = local write "右"(TRUE ("上")) -> ()
                  }
                  frame #1 {
                    n145 = Wait (ms)(milliseconds to wait=u32 60 ("等待时间（毫秒）")) -> ()  [unwired: 1 out]
                  }
                  frame #2 {
                    n146 = local write "右"(FALSE ("上")) -> ()
                  }
                  frame #3 {
                    n147 = Wait (ms)(milliseconds to wait=u32 60 ("等待时间（毫秒）")) -> ()  [unwired: 1 out]
                  }
                }
              }
              frame "Down" {
                n148 = stacked-sequence {
                  frame #0 {
                    n149 = local write "下"(TRUE ("上")) -> ()
                  }
                  frame #1 {
                    n150 = Wait (ms)(milliseconds to wait=u32 60 ("等待时间（毫秒）")) -> ()  [unwired: 1 out]
                  }
                  frame #2 {
                    n151 = local write "下"(FALSE ("上")) -> ()
                  }
                  frame #3 {
                    n152 = Wait (ms)(milliseconds to wait=u32 60 ("等待时间（毫秒）")) -> ()  [unwired: 1 out]
                  }
                }
              }
              frame "Left" {
                n153 = stacked-sequence {
                  frame #0 {
                    n154 = local write "左"(TRUE ("上")) -> ()
                  }
                  frame #1 {
                    n155 = Wait (ms)(milliseconds to wait=u32 60 ("等待时间（毫秒）")) -> ()  [unwired: 1 out]
                  }
                  frame #2 {
                    n156 = local write "左"(FALSE ("上")) -> ()
                  }
                  frame #3 {
                    n157 = Wait (ms)(milliseconds to wait=u32 60 ("等待时间（毫秒）")) -> ()  [unwired: 1 out]
                  }
                }
              }
            }
          }
          event "下": Mouse Down {
            n158 = event-data() -> ()  [unwired: 1 in, 8 out]
            n159 = stacked-sequence {
              frame #0 {
                n160 = local write "下"(TRUE ("上")) -> ()
              }
              frame #1 {
                n161 = Wait (ms)(milliseconds to wait=u32 60 ("等待时间（毫秒）")) -> ()  [unwired: 1 out]
              }
              frame #2 {
                n162 = local write "下"(FALSE ("上")) -> ()
              }
              frame #3 {
                n163 = Wait (ms)(milliseconds to wait=u32 60 ("等待时间（毫秒）")) -> ()  [unwired: 1 out]
              }
            }
          }
          event "存档": Mouse Down {
            n164 = event-data() -> ()  [unwired: 1 in, 8 out]
          }
          event "读档": Value Change {
            n165 = event-data() -> ()  [unwired: 1 in, 6 out]
          }
          event "右": Mouse Down {
            n166 = event-data() -> ()  [unwired: 1 in, 8 out]
            n167 = stacked-sequence {
              frame #0 {
                n168 = local write "右"(TRUE ("上")) -> ()
              }
              frame #1 {
                n169 = Wait (ms)(milliseconds to wait=u32 60 ("等待时间（毫秒）")) -> ()  [unwired: 1 out]
              }
              frame #2 {
                n170 = local write "右"(FALSE ("上")) -> ()
              }
              frame #3 {
                n171 = Wait (ms)(milliseconds to wait=u32 60 ("等待时间（毫秒）")) -> ()  [unwired: 1 out]
              }
            }
          }
          event "左": Mouse Down {
            n172 = event-data() -> ()  [unwired: 1 in, 8 out]
            n173 = stacked-sequence {
              frame #0 {
                n174 = local write "左"(TRUE ("上")) -> ()
              }
              frame #1 {
                n175 = Wait (ms)(milliseconds to wait=u32 60 ("等待时间（毫秒）")) -> ()  [unwired: 1 out]
              }
              frame #2 {
                n176 = local write "左"(FALSE ("上")) -> ()
              }
              frame #3 {
                n177 = Wait (ms)(milliseconds to wait=u32 60 ("等待时间（毫秒）")) -> ()  [unwired: 1 out]
              }
            }
          }
          event Timeout {
            w441 = FALSE
            n178 = event-data() -> ()  [unwired: 1 in, 3 out]
            n179 = local write "上"(w441) -> ()
            n180 = local write "左"(w441) -> ()
            n181 = local write "右"(w441) -> ()
            n182 = local write "下"(w441) -> ()
          }
          event "时间到": Value Change {
            n183 = event-data() -> ()  [unwired: 1 in, 6 out]
          }
        }
        n184 = case shown="\"绿\"" w326 {
          tunnel: w325 -> [_ _ _ _ w356 w364 w372 w382]
          tunnel: w323 -> [_ w347 w350 _ w353 w361 w369 w377]
          tunnel: [w343 w347 w350 w352 w355 w363 w371 w379] -> w322
          tunnel: [w343 0 0 w352 w353 w361 w369 w377] -> w321
          tunnel: ["Game: Read" "Game: Save" "Game: Option" "Game: Exit" w354 w362 w370 w378] -> w318
          frame "读档" {
            w343 = 0
          }
          frame "存档" {
          }
          frame "按错", Default {
          }
          frame "退出" {
            w352 = 0
          }
          frame "黄" {
            n185 = Equal?(x=w356, y=u64 3) -> (x = y?=w358:bool)
            n186 = case shown="真" w358 {
              tunnel: ["Game: Exit" "Game: Option"] -> w354
              frame False {
              }
              frame True {
              }
            }
            n187 = Increment(x=w353) -> (x+1=w355:i32)
          }
          frame "红" {
            n188 = Equal?(x=w364, y=u64 2) -> (x = y?=w366:bool)
            n189 = case shown="假" w366 {
              tunnel: ["Game: Exit" "Game: Option"] -> w362
              frame False {
              }
              frame True {
              }
            }
            n190 = Increment(x=w361) -> (x+1=w363:i32)
          }
          frame "蓝" {
            n191 = Equal?(x=w372, y=u64 1) -> (x = y?=w374:bool)
            n192 = case shown="真" w374 {
              tunnel: ["Game: Exit" "Game: Option"] -> w370
              frame False {
              }
              frame True {
              }
            }
            n193 = Increment(x=w369) -> (x+1=w371:i32)
          }
          frame "绿" {
            n194 = Equal?(x=w382, y=u64 0) -> (x = y?=w381:bool)
            n195 = case shown="真" w381 {
              tunnel: ["Game: Exit" "Game: Option"] -> w378
              frame False {
              }
              frame True {
              }
            }
            n196 = Increment(x=w377) -> (x+1=w379:i32)
          }
        }
        n197 = local read "亮灯次数"() -> (w320:i32)
        n198 = Greater Or Equal?(x=w321, y=w320) -> (x >= y?=w317:bool)
        n199 = local read "时间到"() -> (w319:bool)
        n200 = case shown="假" w319 {
          tunnel: w318 -> [w333 _]
          tunnel: w317 -> [w332 _]
          tunnel: [w331 "Game: Exit"] -> w316
          frame False {
            n201 = case shown="\"Game: Option\", 默认" w333 {
              selector: w333 -> [w335 w339 w340 w341]
              tunnel: w332 -> [w336 _ _ _]
              tunnel: [w334 w339 w340 w341] -> w331
              frame "Game: Option", Default {
                n202 = case shown="真" w336 {
                  tunnel: [w337 "Game: stop counting"] -> w334
                  tunnel: w335 -> [w337 _]
                  frame False {
                  }
                  frame True {
                  }
                }
              }
              frame "Game: Read" {
              }
              frame "Game: Save" {
              }
              frame "Game: Exit" {
              }
            }
          }
          frame True {
          }
        }
        n203 = call <vilib>:"Add State(s) to Queue__JKI_lib_State_Machine.vi"("State(s) in (\"\")"=w330, "State(s) at Back (\"\")"=w316) -> ("States Out"=w329:string)  [unwired: 13 in]
      }
      frame "Game: Exit" {
        # "Template Separator\n(You can make a copy of, or modify, this frame)"
        n204 = local read "难度"() -> (w447:string)
        n205 = local read "分数"() -> (w452:i32)
        n206 = flat-sequence {
          frame #0 {
            # "延时确保倒计时结束"
            n207 = local write "结束"(TRUE ("停止计时")) -> ()
            n208 = Wait (ms)(milliseconds to wait=u32 5 ("等待时间（毫秒）")) -> ()  [unwired: 1 out]
          }
        }
        n209 = Number To Decimal String(number=w452) -> (decimal integer string=w444:string)  [unwired: 1 in]
        n210 = Concatenate Strings("游戏结束！", "\n", "难度：" ("字符串"), w447, "\n", "得分：" ("字符串"), w444) -> (w451:string)
        n211 = One Button Dialog(message=w451) -> ()  [unwired: 1 in, 1 out]
        n212 = call <vilib>:"Add State(s) to Queue__JKI_lib_State_Machine.vi"("State(s) in (\"\")"=w460, "State(s) at Back (\"\")"="Game: Exit" ("State(s) at Back (\"\")")) -> ("States Out"=w459:string)  [unwired: 13 in]
      }
      frame "Game: stop counting" {
        # "Template Separator\n(You can make a copy of, or modify, this frame)"
        n213 = local read "亮灯次数"() -> (w464:i32)
        n214 = local read "分数"() -> (w465:i32)
        n215 = Increment(x=w465) -> (x+1=w463:i32)
        n216 = Increment(x=w464) -> (x+1=w466:i32)
        n217 = local write "分数"(w463) -> ()
        n218 = local write "是否开始计时？"(FALSE ("是否开始计时？")) -> ()
        n219 = local write "亮灯次数"(w466) -> ()
        n220 = Number To Decimal String(number=w463) -> (decimal integer string=w472:string)  [unwired: 1 in]
        n221 = local read "难度"() -> (w474:string)
        n222 = Bundle By Name(cluster=w468, "Core.积分_保存"=w465, "Core.亮灯次数_保存"=w464) -> (w467:T4)
        n223 = Concatenate Strings(w474, "模式：" ("字符串"), w472, "分" ("字符串")) -> (→"难度：分数":string)
        n224 = Wait (ms)(milliseconds to wait=u32 150 ("等待时间（毫秒）")) -> ()  [unwired: 1 out]
        n225 = call <vilib>:"Add State(s) to Queue__JKI_lib_State_Machine.vi"("State(s) in (\"\")"=w481, "State(s) at Back (\"\")"="Game: Twinkle" ("State(s) at Back (\"\")")) -> ("States Out"=w480:string)  [unwired: 13 in]
      }
    }
  }
  n226 = while "While循环" {
    shift-right: [w487] -> _
    shift-left: enum16{"倒计时", "初始化"}."初始化" -> [w488]
    stop <- w482 stop-if-true
    # "倒计时"
    n227 = local read "亮灯次数"() -> (w484:i32)
    n228 = Increment(x=w484) -> (x+1=w483:i32)
    n229 = local read "超时时间"() -> (w486:i32)
    n230 = Multiply(x=w486, y=w483) -> (x*y=w485:i32)
    n231 = case shown="\"倒计时\"" w488 {
      tunnel: [enum16{"倒计时", "初始化"}."倒计时" enum16{"倒计时", "初始化"}."倒计时"] -> w487
      tunnel: w485 -> [w489 _]
      tunnel: [w490 FALSE] -> w482
      frame "倒计时" {
        n232 = case shown="真" "是否开始计时？" {
          tunnel: w489 -> [_ w497]
          tunnel: [w493 w496] -> w490
          frame False {
            n233 = local read "结束"() -> (w495:bool)
            n234 = Or(x=w495, y=FALSE) -> (x .or. y?=w493:bool)
          }
          frame True {
            n235 = property on="倒计时" class="Slide (严格)"("Scale.Maximum"=w497) -> ()  [unwired: 2 in, 2 out]
            n236 = for {
              N: w497 -> [w508]
              tunnel: [w499] -> w496
              i -> [w509]
              stop <- w502 stop-if-true
              n237 = local read "时间到"() -> (w504:bool)
              n238 = Subtract(x=w508, y=w509) -> (x-y=w506:i32)
              "倒计时" <- w506
              n239 = local read "是否开始计时？"() -> (w505:bool)
              n240 = Less Or Equal?(x=w506, y=1) -> (x <= y?=w500:bool)
              n241 = Not(x=w505) -> (.not. x?=w503:bool)
              n242 = case shown="假" w500 {
                tunnel: w504 -> [_ w511]
                frame False {
                }
                frame True {
                  n243 = case shown="真" w511 {
                    frame False {
                      n244 = property on="时间到" class="Bool (严格)"("Val(Sgnl)"=TRUE ("值(信号)")) -> ()  [unwired: 2 in, 2 out]
                    }
                    frame True {
                      n245 = property on="时间到" class="Bool (严格)"("Val(Sgnl)"=FALSE ("值(信号)")) -> ()  [unwired: 2 in, 2 out]
                    }
                  }
                }
              }
              n246 = local read "结束"() -> (w498:bool)
              n247 = Or(x=w503, y=w500) -> (x .or. y?=w501:bool)
              n248 = Or(x=w501, y=w498) -> (x .or. y?=w502:bool)
              n249 = Or(x=w498, y=w500) -> (x .or. y?=w499:bool)
              n250 = Wait (ms)(milliseconds to wait=u32 1 ("等待时间（毫秒）")) -> ()  [unwired: 1 out]
            }
          }
        }
      }
      frame "初始化", Default {
        n251 = invoke on="是否开始计时？" class="Bool (严格)" method="Reinit To Default"() -> ()  [unwired: 3 in, 3 out]
        n252 = local write "倒计时"(1111111111 ("滑动杆")) -> ()
      }
    }
  }
